vi "InitMeasurement.vi"(8 "error in (no error)":errorcluster) -> (0 "error out":errorcluster)   [LabVIEW 2015, in "ESLSCDLL.lvlib"]
uses:
  ESLSCDLL.lvlib
  Globals.vi
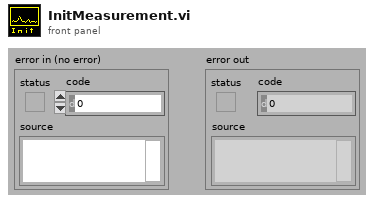
[diagram p1: front panel]
types:
  T1 = cluster{"region size[0]":u32, "region size[1]":u32, "region size[2]":u32, "region size[3]":u32, "region size[4]":u32, "region size[5]":u32, "region size[6]":u32, "region size[7]":u32}
  T2 = cluster{"dac board1[0]":u32, "dac board1[1]":u32, "dac board1[2]":u32, "dac board1[3]":u32, "dac board1[4]":u32, "dac board1[5]":u32, "dac board1[6]":u32, "dac board1[7]":u32}
  T3 = cluster{"ioctrl out width[5ns][0]":u32, "ioctrl out width[5ns][1]":u32, "ioctrl out width[5ns][2]":u32, "ioctrl out width[5ns][3]":u32, "ioctrl out width[5ns][4]":u32, "ioctrl out width[5ns][5]":u32, "ioctrl out width[5ns][6]":u32, "ioctrl out width[5ns][7]":u32}
  T4 = cluster{"ioctrl out delay[5ns][0]":u32, "ioctrl out delay[5ns][1]":u32, "ioctrl out delay[5ns][2]":u32, "ioctrl out delay[5ns][3]":u32, "ioctrl out delay[5ns][4]":u32, "ioctrl out delay[5ns][5]":u32, "ioctrl out delay[5ns][6]":u32, "ioctrl out delay[5ns][7]":u32}
  T5 = cluster{"dac board2[0]":u32, "dac board2[1]":u32, "dac board2[2]":u32, "dac board2[3]":u32, "dac board2[4]":u32, "dac board2[5]":u32, "dac board2[6]":u32, "dac board2[7]":u32}
  T6 = cluster{"[0]":u8, "[1]":u8, "[2]":u8, "[3]":u8, "[4]":u8, "[5]":u8, "[6]":u8, "[7]":u8, "[8]":u8, "[9]":u8, "[10]":u8, "[11]":u8, "[12]":u8, "[13]":u8, "[14]":u8, "[15]":u8, "[16]":u8, "[17]":u8, "[18]":u8, "[19]":u8, "[20]":u8, "[21]":u8, "[22]":u8, "[23]":u8, "[24]":u8, "[25]":u8, "[26]":u8, "[27]":u8, "[28]":u8, "[29]":u8, "[30]":u8, "[31]":u8, "[32]":u8, "[33]":u8, "[34]":u8, "[35]":u8, "[36]":u8, "[37]":u8, "[38]":u8, "[39]":u8, "[40]":u8, "[41]":u8, "[42]":u8, "[43]":u8, "[44]":u8, "[45]":u8, "[46]":u8, "[47]":u8, "[48]":u8, "[49]":u8, "[50]":u8, "[51]":u8, "[52]":u8, "[53]":u8, "[54]":u8, "[55]":u8, "[56]":u8, "[57]":u8, "[58]":u8, "[59]":u8, "[60]":u8, "[61]":u8, "[62]":u8, "[63]":u8, "[64]":u8, "[65]":u8, "[66]":u8, "[67]":u8, "[68]":u8, "[69]":u8, "[70]":u8, "[71]":u8, "[72]":u8, "[73]":u8, "[74]":u8, "[75]":u8, "[76]":u8, "[77]":u8, "[78]":u8, "[79]":u8, "[80]":u8, "[81]":u8, "[82]":u8, "[83]":u8, "[84]":u8, "[85]":u8, "[86]":u8, "[87]":u8, "[88]":u8, "[89]":u8, "[90]":u8, "[91]":u8, "[92]":u8, "[93]":u8, "[94]":u8, "[95]":u8, "[96]":u8, "[97]":u8, "[98]":u8, "[99]":u8, "[100]":u8, "[101]":u8, "[102]":u8, "[103]":u8, "[104]":u8, "[105]":u8, "[106]":u8, "[107]":u8, "[108]":u8, "[109]":u8, "[110]":u8, "[111]":u8, "[112]":u8, "[113]":u8, "[114]":u8, "[115]":u8, "[116]":u8, "[117]":u8, "[118]":u8, "[119]":u8, "[120]":u8, "[121]":u8, "[122]":u8, "[123]":u8, "[124]":u8, "[125]":u8, "[126]":u8, "[127]":u8, "[128]":u8, "[129]":u8, "[130]":u8, "[131]":u8, "[132]":u8, "[133]":u8, "[134]":u8, "[135]":u8, "[136]":u8, "[137]":u8, "[138]":u8, "[139]":u8, "[140]":u8, "[141]":u8, "[142]":u8, "[143]":u8, "[144]":u8, "[145]":u8, "[146]":u8, "[147]":u8, "[148]":u8, "[149]":u8, "[150]":u8, "[151]":u8, "[152]":u8, "[153]":u8, "[154]":u8, "[155]":u8, "[156]":u8, "[157]":u8, "[158]":u8, "[159]":u8, "[160]":u8, "[161]":u8, "[162]":u8, "[163]":u8, "[164]":u8, "[165]":u8, "[166]":u8, "[167]":u8, "[168]":u8, "[169]":u8, "[170]":u8, "[171]":u8, "[172]":u8, "[173]":u8, "[174]":u8, "[175]":u8, "[176]":u8, "[177]":u8, "[178]":u8, "[179]":u8, "[180]":u8, "[181]":u8, "[182]":u8, "[183]":u8, "[184]":u8, "[185]":u8, "[186]":u8, "[187]":u8, "[188]":u8, "[189]":u8, "[190]":u8, "[191]":u8, "[192]":u8, "[193]":u8, "[194]":u8, "[195]":u8, "[196]":u8, "[197]":u8, "[198]":u8, "[199]":u8, "[200]":u8, "[201]":u8, "[202]":u8, "[203]":u8, "[204]":u8, "[205]":u8, "[206]":u8, "[207]":u8, "[208]":u8, "[209]":u8, "[210]":u8, "[211]":u8, "[212]":u8, "[213]":u8, "[214]":u8, "[215]":u8, "[216]":u8, "[217]":u8, "[218]":u8, "[219]":u8, "[220]":u8, "[221]":u8, "[222]":u8, "[223]":u8, "[224]":u8, "[225]":u8, "[226]":u8, "[227]":u8, "[228]":u8, "[229]":u8, "[230]":u8, "[231]":u8, "[232]":u8, "[233]":u8, "[234]":u8, "[235]":u8, "[236]":u8, "[237]":u8, "[238]":u8, "[239]":u8, "[240]":u8, "[241]":u8, "[242]":u8, "[243]":u8, "[244]":u8, "[245]":u8, "[246]":u8, "[247]":u8, "[248]":u8, "[249]":u8, "[250]":u8, "[251]":u8, "[252]":u8, "[253]":u8, "[254]":u8, "[255]":u8}
  T7 = cluster{"dac board3[0]":u32, "dac board3[1]":u32, "dac board3[2]":u32, "dac board3[3]":u32, "dac board3[4]":u32, "dac board3[5]":u32, "dac board3[6]":u32, "dac board3[7]":u32}
  T8 = cluster{"dac board4[0]":u32, "dac board4[1]":u32, "dac board4[2]":u32, "dac board4[3]":u32, "dac board4[4]":u32, "dac board4[5]":u32, "dac board4[6]":u32, "dac board4[7]":u32}
  T9 = cluster{"dac board5[0]":u32, "dac board5[1]":u32, "dac board5[2]":u32, "dac board5[3]":u32, "dac board5[4]":u32, "dac board5[5]":u32, "dac board5[6]":u32, "dac board5[7]":u32}
  T10 = enum32{"Full Binning", "Region of Interest", "Area"}
  T11 = enum32{"XCK", "Reg/OutTrig", "VON", "DMA_Act", "ASLS", "STIMER", "BTIMER", "INTRSR", "S1", "S2", "BON", "MEASUREON", "SDAT", "BDAT", "SSHUT", "BSHUT", "IFC", "DO_CC_I", "EXPOSURE_WINDOW", "TO_CNT_OUT", "SECON", "I", "unused2", "unused3", "unused4", "unused5", "unused6", "unused7", "unused8", "ENFFR", "ENFFW", "ENFFWRPROT"}
  T12 = enum32{"I", "S1", "S2", "S1&S2", "BTimer", "S1 chopper", "S2 chopper", "S1&S2 chopper"}
  T13 = enum32{"I", "S1", "S2", "S2=EN_I", "STimer", "ASL"}
  T14 = cluster{u32, "sti":enum32{"I", "S1", "S2", "S2=EN_I", "STimer", "ASL"}, "bti":enum32{"I", "S1", "S2", "S1&S2", "BTimer", "S1 chopper", "S2 chopper", "S1&S2 chopper"}, u32, u32, "sdat in 10ns":u32, "bdat in 10ns":u32, "st slope":enum32{"pos", "neg", "both"}, "bt slope":enum32{"neg", "pos", "both"}, "xckdly in 10ns":u32, "sec in 10ns":u32, "cc trigger":enum32{"XCK", "Ext. Trig.", "DAT"}, u32, "CAMERA SYSTEM":u32, "CAMCNT":u32, "PIXEL":u32, u32, u32, "sensor gain":u32, "adc gain":u32, "cool level":u32, u32, "gpx offset":u32, "LINES":u32, "VFREQ":u32, "fft mode":enum32{"Full Binning", "Region of Interest", "Area"}, "area lines binning":u32, "nor":u32, u8, "region size":cluster{"region size[0]":u32, "region size[1]":u32, "region size[2]":u32, "region size[3]":u32, "region size[4]":u32, "region size[5]":u32, "region size[6]":u32, "region size[7]":u32}, "dac board1":cluster{"dac board1[0]":u32, "dac board1[1]":u32, "dac board1[2]":u32, "dac board1[3]":u32, "dac board1[4]":u32, "dac board1[5]":u32, "dac board1[6]":u32, "dac board1[7]":u32}, "tor":enum32{"XCK", "Reg/OutTrig", "VON", "DMA_Act", "ASLS", "STIMER", "BTIMER", "INTRSR", "S1", "S2", "BON", "MEASUREON", "SDAT", "BDAT", "SSHUT", "BSHUT", "IFC", "DO_CC_I", "EXPOSURE_WINDOW", "TO_CNT_OUT", "SECON", "I", "unused2", "unused3", "unused4", "unused5", "unused6", "unused7", "unused8", "ENFFR", "ENFFW", "ENFFWRPROT"}, "adc mode":enum16{"normal", "ramp", "custom pattern"}, "custom pattern":u32, "bec in 10\nns":u32, u32, "ioctrl impact start pixel":u32, "ioctrl out width[5ns]":cluster{"ioctrl out width[5ns][0]":u32, "ioctrl out width[5ns][1]":u32, "ioctrl out width[5ns][2]":u32, "ioctrl out width[5ns][3]":u32, "ioctrl out width[5ns][4]":u32, "ioctrl out width[5ns][5]":u32, "ioctrl out width[5ns][6]":u32, "ioctrl out width[5ns][7]":u32}, "ioctrl out delay[5ns]":cluster{"ioctrl out delay[5ns][0]":u32, "ioctrl out delay[5ns][1]":u32, "ioctrl out delay[5ns][2]":u32, "ioctrl out delay[5ns][3]":u32, "ioctrl out delay[5ns][4]":u32, "ioctrl out delay[5ns][5]":u32, "ioctrl out delay[5ns][6]":u32, "ioctrl out delay[5ns][7]":u32}, "ioctrl t0 period[10ns]":u32, "dma buffer size in scans":u32, "tocnt":u32, "ticnt":u32, u32, u32, cluster{"[0]":u8, "[1]":u8, "[2]":u8, "[3]":u8, "[4]":u8, "[5]":u8, "[6]":u8, "[7]":u8, "[8]":u8, "[9]":u8, "[10]":u8, "[11]":u8, "[12]":u8, "[13]":u8, "[14]":u8, "[15]":u8, "[16]":u8, "[17]":u8, "[18]":u8, "[19]":u8, "[20]":u8, "[21]":u8, "[22]":u8, "[23]":u8, "[24]":u8, "[25]":u8, "[26]":u8, "[27]":u8, "[28]":u8, "[29]":u8, "[30]":u8, "[31]":u8, "[32]":u8, "[33]":u8, "[34]":u8, "[35]":u8, "[36]":u8, "[37]":u8, "[38]":u8, "[39]":u8, "[40]":u8, "[41]":u8, "[42]":u8, "[43]":u8, "[44]":u8, "[45]":u8, "[46]":u8, "[47]":u8, "[48]":u8, "[49]":u8, "[50]":u8, "[51]":u8, "[52]":u8, "[53]":u8, "[54]":u8, "[55]":u8, "[56]":u8, "[57]":u8, "[58]":u8, "[59]":u8, "[60]":u8, "[61]":u8, "[62]":u8, "[63]":u8, "[64]":u8, "[65]":u8, "[66]":u8, "[67]":u8, "[68]":u8, "[69]":u8, "[70]":u8, "[71]":u8, "[72]":u8, "[73]":u8, "[74]":u8, "[75]":u8, "[76]":u8, "[77]":u8, "[78]":u8, "[79]":u8, "[80]":u8, "[81]":u8, "[82]":u8, "[83]":u8, "[84]":u8, "[85]":u8, "[86]":u8, "[87]":u8, "[88]":u8, "[89]":u8, "[90]":u8, "[91]":u8, "[92]":u8, "[93]":u8, "[94]":u8, "[95]":u8, "[96]":u8, "[97]":u8, "[98]":u8, "[99]":u8, "[100]":u8, "[101]":u8, "[102]":u8, "[103]":u8, "[104]":u8, "[105]":u8, "[106]":u8, "[107]":u8, "[108]":u8, "[109]":u8, "[110]":u8, "[111]":u8, "[112]":u8, "[113]":u8, "[114]":u8, "[115]":u8, "[116]":u8, "[117]":u8, "[118]":u8, "[119]":u8, "[120]":u8, "[121]":u8, "[122]":u8, "[123]":u8, "[124]":u8, "[125]":u8, "[126]":u8, "[127]":u8, "[128]":u8, "[129]":u8, "[130]":u8, "[131]":u8, "[132]":u8, "[133]":u8, "[134]":u8, "[135]":u8, "[136]":u8, "[137]":u8, "[138]":u8, "[139]":u8, "[140]":u8, "[141]":u8, "[142]":u8, "[143]":u8, "[144]":u8, "[145]":u8, "[146]":u8, "[147]":u8, "[148]":u8, "[149]":u8, "[150]":u8, "[151]":u8, "[152]":u8, "[153]":u8, "[154]":u8, "[155]":u8, "[156]":u8, "[157]":u8, "[158]":u8, "[159]":u8, "[160]":u8, "[161]":u8, "[162]":u8, "[163]":u8, "[164]":u8, "[165]":u8, "[166]":u8, "[167]":u8, "[168]":u8, "[169]":u8, "[170]":u8, "[171]":u8, "[172]":u8, "[173]":u8, "[174]":u8, "[175]":u8, "[176]":u8, "[177]":u8, "[178]":u8, "[179]":u8, "[180]":u8, "[181]":u8, "[182]":u8, "[183]":u8, "[184]":u8, "[185]":u8, "[186]":u8, "[187]":u8, "[188]":u8, "[189]":u8, "[190]":u8, "[191]":u8, "[192]":u8, "[193]":u8, "[194]":u8, "[195]":u8, "[196]":u8, "[197]":u8, "[198]":u8, "[199]":u8, "[200]":u8, "[201]":u8, "[202]":u8, "[203]":u8, "[204]":u8, "[205]":u8, "[206]":u8, "[207]":u8, "[208]":u8, "[209]":u8, "[210]":u8, "[211]":u8, "[212]":u8, "[213]":u8, "[214]":u8, "[215]":u8, "[216]":u8, "[217]":u8, "[218]":u8, "[219]":u8, "[220]":u8, "[221]":u8, "[222]":u8, "[223]":u8, "[224]":u8, "[225]":u8, "[226]":u8, "[227]":u8, "[228]":u8, "[229]":u8, "[230]":u8, "[231]":u8, "[232]":u8, "[233]":u8, "[234]":u8, "[235]":u8, "[236]":u8, "[237]":u8, "[238]":u8, "[239]":u8, "[240]":u8, "[241]":u8, "[242]":u8, "[243]":u8, "[244]":u8, "[245]":u8, "[246]":u8, "[247]":u8, "[248]":u8, "[249]":u8, "[250]":u8, "[251]":u8, "[252]":u8, "[253]":u8, "[254]":u8, "[255]":u8}, "unused (deprecated file split mode)":u32, u32}
  T15 = cluster{u32, "sti":enum32{"I", "S1", "S2", "S2=EN_I", "STimer", "ASL"}, "bti":enum32{"I", "S1", "S2", "S1&S2", "BTimer", "S1 chopper", "S2 chopper", "S1&S2 chopper"}, u32, u32, "sdat in 10ns":u32, "bdat in 10ns":u32, "st slope":enum32{"pos", "neg", "both"}, "bt slope":enum32{"neg", "pos", "both"}, "xckdly in 10ns":u32, "sec in 10ns":u32, "cc trigger":enum32{"XCK", "Ext. Trig.", "DAT"}, u32, "CAMERA SYSTEM":u32, "CAMCNT":u32, "PIXEL":u32, u32, u32, "sensor gain":u32, "adc gain":u32, "cool level":u32, u32, "gpx offset":u32, "LINES":u32, "VFREQ":u32, "fft mode":enum32{"Full Binning", "Region of Interest", "Area"}, "area lines binning":u32, "nor":u32, u8, "region size":cluster{"region size[0]":u32, "region size[1]":u32, "region size[2]":u32, "region size[3]":u32, "region size[4]":u32, "region size[5]":u32, "region size[6]":u32, "region size[7]":u32}, "dac board2":cluster{"dac board2[0]":u32, "dac board2[1]":u32, "dac board2[2]":u32, "dac board2[3]":u32, "dac board2[4]":u32, "dac board2[5]":u32, "dac board2[6]":u32, "dac board2[7]":u32}, "tor":enum32{"XCK", "Reg/OutTrig", "VON", "DMA_Act", "ASLS", "STIMER", "BTIMER", "INTRSR", "S1", "S2", "BON", "MEASUREON", "SDAT", "BDAT", "SSHUT", "BSHUT", "IFC", "DO_CC_I", "EXPOSURE_WINDOW", "TO_CNT_OUT", "SECON", "I", "unused2", "unused3", "unused4", "unused5", "unused6", "unused7", "unused8", "ENFFR", "ENFFW", "ENFFWRPROT"}, "adc mode":enum16{"normal", "ramp", "custom pattern"}, "custom pattern":u32, "bec in 10\nns":u32, u32, "ioctrl impact start pixel":u32, "ioctrl out width[5ns]":cluster{"ioctrl out width[5ns][0]":u32, "ioctrl out width[5ns][1]":u32, "ioctrl out width[5ns][2]":u32, "ioctrl out width[5ns][3]":u32, "ioctrl out width[5ns][4]":u32, "ioctrl out width[5ns][5]":u32, "ioctrl out width[5ns][6]":u32, "ioctrl out width[5ns][7]":u32}, "ioctrl out delay[5ns]":cluster{"ioctrl out delay[5ns][0]":u32, "ioctrl out delay[5ns][1]":u32, "ioctrl out delay[5ns][2]":u32, "ioctrl out delay[5ns][3]":u32, "ioctrl out delay[5ns][4]":u32, "ioctrl out delay[5ns][5]":u32, "ioctrl out delay[5ns][6]":u32, "ioctrl out delay[5ns][7]":u32}, "ioctrl t0 period[10ns]":u32, "dma buffer size in scans":u32, "tocnt":u32, "ticnt":u32, u32, u32, cluster{"[0]":u8, "[1]":u8, "[2]":u8, "[3]":u8, "[4]":u8, "[5]":u8, "[6]":u8, "[7]":u8, "[8]":u8, "[9]":u8, "[10]":u8, "[11]":u8, "[12]":u8, "[13]":u8, "[14]":u8, "[15]":u8, "[16]":u8, "[17]":u8, "[18]":u8, "[19]":u8, "[20]":u8, "[21]":u8, "[22]":u8, "[23]":u8, "[24]":u8, "[25]":u8, "[26]":u8, "[27]":u8, "[28]":u8, "[29]":u8, "[30]":u8, "[31]":u8, "[32]":u8, "[33]":u8, "[34]":u8, "[35]":u8, "[36]":u8, "[37]":u8, "[38]":u8, "[39]":u8, "[40]":u8, "[41]":u8, "[42]":u8, "[43]":u8, "[44]":u8, "[45]":u8, "[46]":u8, "[47]":u8, "[48]":u8, "[49]":u8, "[50]":u8, "[51]":u8, "[52]":u8, "[53]":u8, "[54]":u8, "[55]":u8, "[56]":u8, "[57]":u8, "[58]":u8, "[59]":u8, "[60]":u8, "[61]":u8, "[62]":u8, "[63]":u8, "[64]":u8, "[65]":u8, "[66]":u8, "[67]":u8, "[68]":u8, "[69]":u8, "[70]":u8, "[71]":u8, "[72]":u8, "[73]":u8, "[74]":u8, "[75]":u8, "[76]":u8, "[77]":u8, "[78]":u8, "[79]":u8, "[80]":u8, "[81]":u8, "[82]":u8, "[83]":u8, "[84]":u8, "[85]":u8, "[86]":u8, "[87]":u8, "[88]":u8, "[89]":u8, "[90]":u8, "[91]":u8, "[92]":u8, "[93]":u8, "[94]":u8, "[95]":u8, "[96]":u8, "[97]":u8, "[98]":u8, "[99]":u8, "[100]":u8, "[101]":u8, "[102]":u8, "[103]":u8, "[104]":u8, "[105]":u8, "[106]":u8, "[107]":u8, "[108]":u8, "[109]":u8, "[110]":u8, "[111]":u8, "[112]":u8, "[113]":u8, "[114]":u8, "[115]":u8, "[116]":u8, "[117]":u8, "[118]":u8, "[119]":u8, "[120]":u8, "[121]":u8, "[122]":u8, "[123]":u8, "[124]":u8, "[125]":u8, "[126]":u8, "[127]":u8, "[128]":u8, "[129]":u8, "[130]":u8, "[131]":u8, "[132]":u8, "[133]":u8, "[134]":u8, "[135]":u8, "[136]":u8, "[137]":u8, "[138]":u8, "[139]":u8, "[140]":u8, "[141]":u8, "[142]":u8, "[143]":u8, "[144]":u8, "[145]":u8, "[146]":u8, "[147]":u8, "[148]":u8, "[149]":u8, "[150]":u8, "[151]":u8, "[152]":u8, "[153]":u8, "[154]":u8, "[155]":u8, "[156]":u8, "[157]":u8, "[158]":u8, "[159]":u8, "[160]":u8, "[161]":u8, "[162]":u8, "[163]":u8, "[164]":u8, "[165]":u8, "[166]":u8, "[167]":u8, "[168]":u8, "[169]":u8, "[170]":u8, "[171]":u8, "[172]":u8, "[173]":u8, "[174]":u8, "[175]":u8, "[176]":u8, "[177]":u8, "[178]":u8, "[179]":u8, "[180]":u8, "[181]":u8, "[182]":u8, "[183]":u8, "[184]":u8, "[185]":u8, "[186]":u8, "[187]":u8, "[188]":u8, "[189]":u8, "[190]":u8, "[191]":u8, "[192]":u8, "[193]":u8, "[194]":u8, "[195]":u8, "[196]":u8, "[197]":u8, "[198]":u8, "[199]":u8, "[200]":u8, "[201]":u8, "[202]":u8, "[203]":u8, "[204]":u8, "[205]":u8, "[206]":u8, "[207]":u8, "[208]":u8, "[209]":u8, "[210]":u8, "[211]":u8, "[212]":u8, "[213]":u8, "[214]":u8, "[215]":u8, "[216]":u8, "[217]":u8, "[218]":u8, "[219]":u8, "[220]":u8, "[221]":u8, "[222]":u8, "[223]":u8, "[224]":u8, "[225]":u8, "[226]":u8, "[227]":u8, "[228]":u8, "[229]":u8, "[230]":u8, "[231]":u8, "[232]":u8, "[233]":u8, "[234]":u8, "[235]":u8, "[236]":u8, "[237]":u8, "[238]":u8, "[239]":u8, "[240]":u8, "[241]":u8, "[242]":u8, "[243]":u8, "[244]":u8, "[245]":u8, "[246]":u8, "[247]":u8, "[248]":u8, "[249]":u8, "[250]":u8, "[251]":u8, "[252]":u8, "[253]":u8, "[254]":u8, "[255]":u8}, "unused (deprecated file split mode)":u32, u32}
  T16 = cluster{u32, "sti":enum32{"I", "S1", "S2", "S2=EN_I", "STimer", "ASL"}, "bti":enum32{"I", "S1", "S2", "S1&S2", "BTimer", "S1 chopper", "S2 chopper", "S1&S2 chopper"}, u32, u32, "sdat in 10ns":u32, "bdat in 10ns":u32, "st slope":enum32{"pos", "neg", "both"}, "bt slope":enum32{"neg", "pos", "both"}, "xckdly in 10ns":u32, "sec in 10ns":u32, "cc trigger":enum32{"XCK", "Ext. Trig.", "DAT"}, u32, "CAMERA SYSTEM":u32, "CAMCNT":u32, "PIXEL":u32, u32, u32, "sensor gain":u32, "adc gain":u32, "cool level":u32, u32, "gpx offset":u32, "LINES":u32, "VFREQ":u32, "fft mode":enum32{"Full Binning", "Region of Interest", "Area"}, "area lines binning":u32, "nor":u32, u8, "region size":cluster{"region size[0]":u32, "region size[1]":u32, "region size[2]":u32, "region size[3]":u32, "region size[4]":u32, "region size[5]":u32, "region size[6]":u32, "region size[7]":u32}, "dac board3":cluster{"dac board3[0]":u32, "dac board3[1]":u32, "dac board3[2]":u32, "dac board3[3]":u32, "dac board3[4]":u32, "dac board3[5]":u32, "dac board3[6]":u32, "dac board3[7]":u32}, "tor":enum32{"XCK", "Reg/OutTrig", "VON", "DMA_Act", "ASLS", "STIMER", "BTIMER", "INTRSR", "S1", "S2", "BON", "MEASUREON", "SDAT", "BDAT", "SSHUT", "BSHUT", "IFC", "DO_CC_I", "EXPOSURE_WINDOW", "TO_CNT_OUT", "SECON", "I", "unused2", "unused3", "unused4", "unused5", "unused6", "unused7", "unused8", "ENFFR", "ENFFW", "ENFFWRPROT"}, "adc mode":enum16{"normal", "ramp", "custom pattern"}, "custom pattern":u32, "bec in 10\nns":u32, u32, "ioctrl impact start pixel":u32, "ioctrl out width[5ns]":cluster{"ioctrl out width[5ns][0]":u32, "ioctrl out width[5ns][1]":u32, "ioctrl out width[5ns][2]":u32, "ioctrl out width[5ns][3]":u32, "ioctrl out width[5ns][4]":u32, "ioctrl out width[5ns][5]":u32, "ioctrl out width[5ns][6]":u32, "ioctrl out width[5ns][7]":u32}, "ioctrl out delay[5ns]":cluster{"ioctrl out delay[5ns][0]":u32, "ioctrl out delay[5ns][1]":u32, "ioctrl out delay[5ns][2]":u32, "ioctrl out delay[5ns][3]":u32, "ioctrl out delay[5ns][4]":u32, "ioctrl out delay[5ns][5]":u32, "ioctrl out delay[5ns][6]":u32, "ioctrl out delay[5ns][7]":u32}, "ioctrl t0 period[10ns]":u32, "dma buffer size in scans":u32, "tocnt":u32, "ticnt":u32, u32, u32, cluster{"[0]":u8, "[1]":u8, "[2]":u8, "[3]":u8, "[4]":u8, "[5]":u8, "[6]":u8, "[7]":u8, "[8]":u8, "[9]":u8, "[10]":u8, "[11]":u8, "[12]":u8, "[13]":u8, "[14]":u8, "[15]":u8, "[16]":u8, "[17]":u8, "[18]":u8, "[19]":u8, "[20]":u8, "[21]":u8, "[22]":u8, "[23]":u8, "[24]":u8, "[25]":u8, "[26]":u8, "[27]":u8, "[28]":u8, "[29]":u8, "[30]":u8, "[31]":u8, "[32]":u8, "[33]":u8, "[34]":u8, "[35]":u8, "[36]":u8, "[37]":u8, "[38]":u8, "[39]":u8, "[40]":u8, "[41]":u8, "[42]":u8, "[43]":u8, "[44]":u8, "[45]":u8, "[46]":u8, "[47]":u8, "[48]":u8, "[49]":u8, "[50]":u8, "[51]":u8, "[52]":u8, "[53]":u8, "[54]":u8, "[55]":u8, "[56]":u8, "[57]":u8, "[58]":u8, "[59]":u8, "[60]":u8, "[61]":u8, "[62]":u8, "[63]":u8, "[64]":u8, "[65]":u8, "[66]":u8, "[67]":u8, "[68]":u8, "[69]":u8, "[70]":u8, "[71]":u8, "[72]":u8, "[73]":u8, "[74]":u8, "[75]":u8, "[76]":u8, "[77]":u8, "[78]":u8, "[79]":u8, "[80]":u8, "[81]":u8, "[82]":u8, "[83]":u8, "[84]":u8, "[85]":u8, "[86]":u8, "[87]":u8, "[88]":u8, "[89]":u8, "[90]":u8, "[91]":u8, "[92]":u8, "[93]":u8, "[94]":u8, "[95]":u8, "[96]":u8, "[97]":u8, "[98]":u8, "[99]":u8, "[100]":u8, "[101]":u8, "[102]":u8, "[103]":u8, "[104]":u8, "[105]":u8, "[106]":u8, "[107]":u8, "[108]":u8, "[109]":u8, "[110]":u8, "[111]":u8, "[112]":u8, "[113]":u8, "[114]":u8, "[115]":u8, "[116]":u8, "[117]":u8, "[118]":u8, "[119]":u8, "[120]":u8, "[121]":u8, "[122]":u8, "[123]":u8, "[124]":u8, "[125]":u8, "[126]":u8, "[127]":u8, "[128]":u8, "[129]":u8, "[130]":u8, "[131]":u8, "[132]":u8, "[133]":u8, "[134]":u8, "[135]":u8, "[136]":u8, "[137]":u8, "[138]":u8, "[139]":u8, "[140]":u8, "[141]":u8, "[142]":u8, "[143]":u8, "[144]":u8, "[145]":u8, "[146]":u8, "[147]":u8, "[148]":u8, "[149]":u8, "[150]":u8, "[151]":u8, "[152]":u8, "[153]":u8, "[154]":u8, "[155]":u8, "[156]":u8, "[157]":u8, "[158]":u8, "[159]":u8, "[160]":u8, "[161]":u8, "[162]":u8, "[163]":u8, "[164]":u8, "[165]":u8, "[166]":u8, "[167]":u8, "[168]":u8, "[169]":u8, "[170]":u8, "[171]":u8, "[172]":u8, "[173]":u8, "[174]":u8, "[175]":u8, "[176]":u8, "[177]":u8, "[178]":u8, "[179]":u8, "[180]":u8, "[181]":u8, "[182]":u8, "[183]":u8, "[184]":u8, "[185]":u8, "[186]":u8, "[187]":u8, "[188]":u8, "[189]":u8, "[190]":u8, "[191]":u8, "[192]":u8, "[193]":u8, "[194]":u8, "[195]":u8, "[196]":u8, "[197]":u8, "[198]":u8, "[199]":u8, "[200]":u8, "[201]":u8, "[202]":u8, "[203]":u8, "[204]":u8, "[205]":u8, "[206]":u8, "[207]":u8, "[208]":u8, "[209]":u8, "[210]":u8, "[211]":u8, "[212]":u8, "[213]":u8, "[214]":u8, "[215]":u8, "[216]":u8, "[217]":u8, "[218]":u8, "[219]":u8, "[220]":u8, "[221]":u8, "[222]":u8, "[223]":u8, "[224]":u8, "[225]":u8, "[226]":u8, "[227]":u8, "[228]":u8, "[229]":u8, "[230]":u8, "[231]":u8, "[232]":u8, "[233]":u8, "[234]":u8, "[235]":u8, "[236]":u8, "[237]":u8, "[238]":u8, "[239]":u8, "[240]":u8, "[241]":u8, "[242]":u8, "[243]":u8, "[244]":u8, "[245]":u8, "[246]":u8, "[247]":u8, "[248]":u8, "[249]":u8, "[250]":u8, "[251]":u8, "[252]":u8, "[253]":u8, "[254]":u8, "[255]":u8}, "unused (deprecated file split mode)":u32, u32}
  T17 = cluster{u32, "sti":enum32{"I", "S1", "S2", "S2=EN_I", "STimer", "ASL"}, "bti":enum32{"I", "S1", "S2", "S1&S2", "BTimer", "S1 chopper", "S2 chopper", "S1&S2 chopper"}, u32, u32, "sdat in 10ns":u32, "bdat in 10ns":u32, "st slope":enum32{"pos", "neg", "both"}, "bt slope":enum32{"neg", "pos", "both"}, "xckdly in 10ns":u32, "sec in 10ns":u32, "cc trigger":enum32{"XCK", "Ext. Trig.", "DAT"}, u32, "CAMERA SYSTEM":u32, "CAMCNT":u32, "PIXEL":u32, u32, u32, "sensor gain":u32, "adc gain":u32, "cool level":u32, u32, "gpx offset":u32, "LINES":u32, "VFREQ":u32, "fft mode":enum32{"Full Binning", "Region of Interest", "Area"}, "area lines binning":u32, "nor":u32, u8, "region size":cluster{"region size[0]":u32, "region size[1]":u32, "region size[2]":u32, "region size[3]":u32, "region size[4]":u32, "region size[5]":u32, "region size[6]":u32, "region size[7]":u32}, "dac board4":cluster{"dac board4[0]":u32, "dac board4[1]":u32, "dac board4[2]":u32, "dac board4[3]":u32, "dac board4[4]":u32, "dac board4[5]":u32, "dac board4[6]":u32, "dac board4[7]":u32}, "tor":enum32{"XCK", "Reg/OutTrig", "VON", "DMA_Act", "ASLS", "STIMER", "BTIMER", "INTRSR", "S1", "S2", "BON", "MEASUREON", "SDAT", "BDAT", "SSHUT", "BSHUT", "IFC", "DO_CC_I", "EXPOSURE_WINDOW", "TO_CNT_OUT", "SECON", "I", "unused2", "unused3", "unused4", "unused5", "unused6", "unused7", "unused8", "ENFFR", "ENFFW", "ENFFWRPROT"}, "adc mode":enum16{"normal", "ramp", "custom pattern"}, "custom pattern":u32, "bec in 10\nns":u32, u32, "ioctrl impact start pixel":u32, "ioctrl out width[5ns]":cluster{"ioctrl out width[5ns][0]":u32, "ioctrl out width[5ns][1]":u32, "ioctrl out width[5ns][2]":u32, "ioctrl out width[5ns][3]":u32, "ioctrl out width[5ns][4]":u32, "ioctrl out width[5ns][5]":u32, "ioctrl out width[5ns][6]":u32, "ioctrl out width[5ns][7]":u32}, "ioctrl out delay[5ns]":cluster{"ioctrl out delay[5ns][0]":u32, "ioctrl out delay[5ns][1]":u32, "ioctrl out delay[5ns][2]":u32, "ioctrl out delay[5ns][3]":u32, "ioctrl out delay[5ns][4]":u32, "ioctrl out delay[5ns][5]":u32, "ioctrl out delay[5ns][6]":u32, "ioctrl out delay[5ns][7]":u32}, "ioctrl t0 period[10ns]":u32, "dma buffer size in scans":u32, "tocnt":u32, "ticnt":u32, u32, u32, cluster{"[0]":u8, "[1]":u8, "[2]":u8, "[3]":u8, "[4]":u8, "[5]":u8, "[6]":u8, "[7]":u8, "[8]":u8, "[9]":u8, "[10]":u8, "[11]":u8, "[12]":u8, "[13]":u8, "[14]":u8, "[15]":u8, "[16]":u8, "[17]":u8, "[18]":u8, "[19]":u8, "[20]":u8, "[21]":u8, "[22]":u8, "[23]":u8, "[24]":u8, "[25]":u8, "[26]":u8, "[27]":u8, "[28]":u8, "[29]":u8, "[30]":u8, "[31]":u8, "[32]":u8, "[33]":u8, "[34]":u8, "[35]":u8, "[36]":u8, "[37]":u8, "[38]":u8, "[39]":u8, "[40]":u8, "[41]":u8, "[42]":u8, "[43]":u8, "[44]":u8, "[45]":u8, "[46]":u8, "[47]":u8, "[48]":u8, "[49]":u8, "[50]":u8, "[51]":u8, "[52]":u8, "[53]":u8, "[54]":u8, "[55]":u8, "[56]":u8, "[57]":u8, "[58]":u8, "[59]":u8, "[60]":u8, "[61]":u8, "[62]":u8, "[63]":u8, "[64]":u8, "[65]":u8, "[66]":u8, "[67]":u8, "[68]":u8, "[69]":u8, "[70]":u8, "[71]":u8, "[72]":u8, "[73]":u8, "[74]":u8, "[75]":u8, "[76]":u8, "[77]":u8, "[78]":u8, "[79]":u8, "[80]":u8, "[81]":u8, "[82]":u8, "[83]":u8, "[84]":u8, "[85]":u8, "[86]":u8, "[87]":u8, "[88]":u8, "[89]":u8, "[90]":u8, "[91]":u8, "[92]":u8, "[93]":u8, "[94]":u8, "[95]":u8, "[96]":u8, "[97]":u8, "[98]":u8, "[99]":u8, "[100]":u8, "[101]":u8, "[102]":u8, "[103]":u8, "[104]":u8, "[105]":u8, "[106]":u8, "[107]":u8, "[108]":u8, "[109]":u8, "[110]":u8, "[111]":u8, "[112]":u8, "[113]":u8, "[114]":u8, "[115]":u8, "[116]":u8, "[117]":u8, "[118]":u8, "[119]":u8, "[120]":u8, "[121]":u8, "[122]":u8, "[123]":u8, "[124]":u8, "[125]":u8, "[126]":u8, "[127]":u8, "[128]":u8, "[129]":u8, "[130]":u8, "[131]":u8, "[132]":u8, "[133]":u8, "[134]":u8, "[135]":u8, "[136]":u8, "[137]":u8, "[138]":u8, "[139]":u8, "[140]":u8, "[141]":u8, "[142]":u8, "[143]":u8, "[144]":u8, "[145]":u8, "[146]":u8, "[147]":u8, "[148]":u8, "[149]":u8, "[150]":u8, "[151]":u8, "[152]":u8, "[153]":u8, "[154]":u8, "[155]":u8, "[156]":u8, "[157]":u8, "[158]":u8, "[159]":u8, "[160]":u8, "[161]":u8, "[162]":u8, "[163]":u8, "[164]":u8, "[165]":u8, "[166]":u8, "[167]":u8, "[168]":u8, "[169]":u8, "[170]":u8, "[171]":u8, "[172]":u8, "[173]":u8, "[174]":u8, "[175]":u8, "[176]":u8, "[177]":u8, "[178]":u8, "[179]":u8, "[180]":u8, "[181]":u8, "[182]":u8, "[183]":u8, "[184]":u8, "[185]":u8, "[186]":u8, "[187]":u8, "[188]":u8, "[189]":u8, "[190]":u8, "[191]":u8, "[192]":u8, "[193]":u8, "[194]":u8, "[195]":u8, "[196]":u8, "[197]":u8, "[198]":u8, "[199]":u8, "[200]":u8, "[201]":u8, "[202]":u8, "[203]":u8, "[204]":u8, "[205]":u8, "[206]":u8, "[207]":u8, "[208]":u8, "[209]":u8, "[210]":u8, "[211]":u8, "[212]":u8, "[213]":u8, "[214]":u8, "[215]":u8, "[216]":u8, "[217]":u8, "[218]":u8, "[219]":u8, "[220]":u8, "[221]":u8, "[222]":u8, "[223]":u8, "[224]":u8, "[225]":u8, "[226]":u8, "[227]":u8, "[228]":u8, "[229]":u8, "[230]":u8, "[231]":u8, "[232]":u8, "[233]":u8, "[234]":u8, "[235]":u8, "[236]":u8, "[237]":u8, "[238]":u8, "[239]":u8, "[240]":u8, "[241]":u8, "[242]":u8, "[243]":u8, "[244]":u8, "[245]":u8, "[246]":u8, "[247]":u8, "[248]":u8, "[249]":u8, "[250]":u8, "[251]":u8, "[252]":u8, "[253]":u8, "[254]":u8, "[255]":u8}, "unused (deprecated file split mode)":u32, u32}
  T18 = cluster{u32, "sti":enum32{"I", "S1", "S2", "S2=EN_I", "STimer", "ASL"}, "bti":enum32{"I", "S1", "S2", "S1&S2", "BTimer", "S1 chopper", "S2 chopper", "S1&S2 chopper"}, u32, u32, "sdat in 10ns":u32, "bdat in 10ns":u32, "st slope":enum32{"pos", "neg", "both"}, "bt slope":enum32{"neg", "pos", "both"}, "xckdly in 10ns":u32, "sec in 10ns":u32, "cc trigger":enum32{"XCK", "Ext. Trig.", "DAT"}, u32, "CAMERA SYSTEM":u32, "CAMCNT":u32, "PIXEL":u32, u32, u32, "sensor gain":u32, "adc gain":u32, "cool level":u32, u32, "gpx offset":u32, "LINES":u32, "VFREQ":u32, "fft mode":enum32{"Full Binning", "Region of Interest", "Area"}, "area lines binning":u32, "nor":u32, u8, "region size":cluster{"region size[0]":u32, "region size[1]":u32, "region size[2]":u32, "region size[3]":u32, "region size[4]":u32, "region size[5]":u32, "region size[6]":u32, "region size[7]":u32}, "dac board5":cluster{"dac board5[0]":u32, "dac board5[1]":u32, "dac board5[2]":u32, "dac board5[3]":u32, "dac board5[4]":u32, "dac board5[5]":u32, "dac board5[6]":u32, "dac board5[7]":u32}, "tor":enum32{"XCK", "Reg/OutTrig", "VON", "DMA_Act", "ASLS", "STIMER", "BTIMER", "INTRSR", "S1", "S2", "BON", "MEASUREON", "SDAT", "BDAT", "SSHUT", "BSHUT", "IFC", "DO_CC_I", "EXPOSURE_WINDOW", "TO_CNT_OUT", "SECON", "I", "unused2", "unused3", "unused4", "unused5", "unused6", "unused7", "unused8", "ENFFR", "ENFFW", "ENFFWRPROT"}, "adc mode":enum16{"normal", "ramp", "custom pattern"}, "custom pattern":u32, "bec in 10\nns":u32, u32, "ioctrl impact start pixel":u32, "ioctrl out width[5ns]":cluster{"ioctrl out width[5ns][0]":u32, "ioctrl out width[5ns][1]":u32, "ioctrl out width[5ns][2]":u32, "ioctrl out width[5ns][3]":u32, "ioctrl out width[5ns][4]":u32, "ioctrl out width[5ns][5]":u32, "ioctrl out width[5ns][6]":u32, "ioctrl out width[5ns][7]":u32}, "ioctrl out delay[5ns]":cluster{"ioctrl out delay[5ns][0]":u32, "ioctrl out delay[5ns][1]":u32, "ioctrl out delay[5ns][2]":u32, "ioctrl out delay[5ns][3]":u32, "ioctrl out delay[5ns][4]":u32, "ioctrl out delay[5ns][5]":u32, "ioctrl out delay[5ns][6]":u32, "ioctrl out delay[5ns][7]":u32}, "ioctrl t0 period[10ns]":u32, "dma buffer size in scans":u32, "tocnt":u32, "ticnt":u32, u32, u32, cluster{"[0]":u8, "[1]":u8, "[2]":u8, "[3]":u8, "[4]":u8, "[5]":u8, "[6]":u8, "[7]":u8, "[8]":u8, "[9]":u8, "[10]":u8, "[11]":u8, "[12]":u8, "[13]":u8, "[14]":u8, "[15]":u8, "[16]":u8, "[17]":u8, "[18]":u8, "[19]":u8, "[20]":u8, "[21]":u8, "[22]":u8, "[23]":u8, "[24]":u8, "[25]":u8, "[26]":u8, "[27]":u8, "[28]":u8, "[29]":u8, "[30]":u8, "[31]":u8, "[32]":u8, "[33]":u8, "[34]":u8, "[35]":u8, "[36]":u8, "[37]":u8, "[38]":u8, "[39]":u8, "[40]":u8, "[41]":u8, "[42]":u8, "[43]":u8, "[44]":u8, "[45]":u8, "[46]":u8, "[47]":u8, "[48]":u8, "[49]":u8, "[50]":u8, "[51]":u8, "[52]":u8, "[53]":u8, "[54]":u8, "[55]":u8, "[56]":u8, "[57]":u8, "[58]":u8, "[59]":u8, "[60]":u8, "[61]":u8, "[62]":u8, "[63]":u8, "[64]":u8, "[65]":u8, "[66]":u8, "[67]":u8, "[68]":u8, "[69]":u8, "[70]":u8, "[71]":u8, "[72]":u8, "[73]":u8, "[74]":u8, "[75]":u8, "[76]":u8, "[77]":u8, "[78]":u8, "[79]":u8, "[80]":u8, "[81]":u8, "[82]":u8, "[83]":u8, "[84]":u8, "[85]":u8, "[86]":u8, "[87]":u8, "[88]":u8, "[89]":u8, "[90]":u8, "[91]":u8, "[92]":u8, "[93]":u8, "[94]":u8, "[95]":u8, "[96]":u8, "[97]":u8, "[98]":u8, "[99]":u8, "[100]":u8, "[101]":u8, "[102]":u8, "[103]":u8, "[104]":u8, "[105]":u8, "[106]":u8, "[107]":u8, "[108]":u8, "[109]":u8, "[110]":u8, "[111]":u8, "[112]":u8, "[113]":u8, "[114]":u8, "[115]":u8, "[116]":u8, "[117]":u8, "[118]":u8, "[119]":u8, "[120]":u8, "[121]":u8, "[122]":u8, "[123]":u8, "[124]":u8, "[125]":u8, "[126]":u8, "[127]":u8, "[128]":u8, "[129]":u8, "[130]":u8, "[131]":u8, "[132]":u8, "[133]":u8, "[134]":u8, "[135]":u8, "[136]":u8, "[137]":u8, "[138]":u8, "[139]":u8, "[140]":u8, "[141]":u8, "[142]":u8, "[143]":u8, "[144]":u8, "[145]":u8, "[146]":u8, "[147]":u8, "[148]":u8, "[149]":u8, "[150]":u8, "[151]":u8, "[152]":u8, "[153]":u8, "[154]":u8, "[155]":u8, "[156]":u8, "[157]":u8, "[158]":u8, "[159]":u8, "[160]":u8, "[161]":u8, "[162]":u8, "[163]":u8, "[164]":u8, "[165]":u8, "[166]":u8, "[167]":u8, "[168]":u8, "[169]":u8, "[170]":u8, "[171]":u8, "[172]":u8, "[173]":u8, "[174]":u8, "[175]":u8, "[176]":u8, "[177]":u8, "[178]":u8, "[179]":u8, "[180]":u8, "[181]":u8, "[182]":u8, "[183]":u8, "[184]":u8, "[185]":u8, "[186]":u8, "[187]":u8, "[188]":u8, "[189]":u8, "[190]":u8, "[191]":u8, "[192]":u8, "[193]":u8, "[194]":u8, "[195]":u8, "[196]":u8, "[197]":u8, "[198]":u8, "[199]":u8, "[200]":u8, "[201]":u8, "[202]":u8, "[203]":u8, "[204]":u8, "[205]":u8, "[206]":u8, "[207]":u8, "[208]":u8, "[209]":u8, "[210]":u8, "[211]":u8, "[212]":u8, "[213]":u8, "[214]":u8, "[215]":u8, "[216]":u8, "[217]":u8, "[218]":u8, "[219]":u8, "[220]":u8, "[221]":u8, "[222]":u8, "[223]":u8, "[224]":u8, "[225]":u8, "[226]":u8, "[227]":u8, "[228]":u8, "[229]":u8, "[230]":u8, "[231]":u8, "[232]":u8, "[233]":u8, "[234]":u8, "[235]":u8, "[236]":u8, "[237]":u8, "[238]":u8, "[239]":u8, "[240]":u8, "[241]":u8, "[242]":u8, "[243]":u8, "[244]":u8, "[245]":u8, "[246]":u8, "[247]":u8, "[248]":u8, "[249]":u8, "[250]":u8, "[251]":u8, "[252]":u8, "[253]":u8, "[254]":u8, "[255]":u8}, "unused (deprecated file split mode)":u32, u32}
  T19 = cluster{"board_sel":u32, "nos":u32, "nob":u32, u32, "cont pause in microseconds":u32, cluster{u32, "sti":enum32{"I", "S1", "S2", "S2=EN_I", "STimer", "ASL"}, "bti":enum32{"I", "S1", "S2", "S1&S2", "BTimer", "S1 chopper", "S2 chopper", "S1&S2 chopper"}, u32, u32, "sdat in 10ns":u32, "bdat in 10ns":u32, "st slope":enum32{"pos", "neg", "both"}, "bt slope":enum32{"neg", "pos", "both"}, "xckdly in 10ns":u32, "sec in 10ns":u32, "cc trigger":enum32{"XCK", "Ext. Trig.", "DAT"}, u32, "CAMERA SYSTEM":u32, "CAMCNT":u32, "PIXEL":u32, u32, u32, "sensor gain":u32, "adc gain":u32, "cool level":u32, u32, "gpx offset":u32, "LINES":u32, "VFREQ":u32, "fft mode":enum32{"Full Binning", "Region of Interest", "Area"}, "area lines binning":u32, "nor":u32, u8, "region size":cluster{"region size[0]":u32, "region size[1]":u32, "region size[2]":u32, "region size[3]":u32, "region size[4]":u32, "region size[5]":u32, "region size[6]":u32, "region size[7]":u32}, "dac board1":cluster{"dac board1[0]":u32, "dac board1[1]":u32, "dac board1[2]":u32, "dac board1[3]":u32, "dac board1[4]":u32, "dac board1[5]":u32, "dac board1[6]":u32, "dac board1[7]":u32}, "tor":enum32{"XCK", "Reg/OutTrig", "VON", "DMA_Act", "ASLS", "STIMER", "BTIMER", "INTRSR", "S1", "S2", "BON", "MEASUREON", "SDAT", "BDAT", "SSHUT", "BSHUT", "IFC", "DO_CC_I", "EXPOSURE_WINDOW", "TO_CNT_OUT", "SECON", "I", "unused2", "unused3", "unused4", "unused5", "unused6", "unused7", "unused8", "ENFFR", "ENFFW", "ENFFWRPROT"}, "adc mode":enum16{"normal", "ramp", "custom pattern"}, "custom pattern":u32, "bec in 10\nns":u32, u32, "ioctrl impact start pixel":u32, "ioctrl out width[5ns]":cluster{"ioctrl out width[5ns][0]":u32, "ioctrl out width[5ns][1]":u32, "ioctrl out width[5ns][2]":u32, "ioctrl out width[5ns][3]":u32, "ioctrl out width[5ns][4]":u32, "ioctrl out width[5ns][5]":u32, "ioctrl out width[5ns][6]":u32, "ioctrl out width[5ns][7]":u32}, "ioctrl out delay[5ns]":cluster{"ioctrl out delay[5ns][0]":u32, "ioctrl out delay[5ns][1]":u32, "ioctrl out delay[5ns][2]":u32, "ioctrl out delay[5ns][3]":u32, "ioctrl out delay[5ns][4]":u32, "ioctrl out delay[5ns][5]":u32, "ioctrl out delay[5ns][6]":u32, "ioctrl out delay[5ns][7]":u32}, "ioctrl t0 period[10ns]":u32, "dma buffer size in scans":u32, "tocnt":u32, "ticnt":u32, u32, u32, cluster{"[0]":u8, "[1]":u8, "[2]":u8, "[3]":u8, "[4]":u8, "[5]":u8, "[6]":u8, "[7]":u8, "[8]":u8, "[9]":u8, "[10]":u8, "[11]":u8, "[12]":u8, "[13]":u8, "[14]":u8, "[15]":u8, "[16]":u8, "[17]":u8, "[18]":u8, "[19]":u8, "[20]":u8, "[21]":u8, "[22]":u8, "[23]":u8, "[24]":u8, "[25]":u8, "[26]":u8, "[27]":u8, "[28]":u8, "[29]":u8, "[30]":u8, "[31]":u8, "[32]":u8, "[33]":u8, "[34]":u8, "[35]":u8, "[36]":u8, "[37]":u8, "[38]":u8, "[39]":u8, "[40]":u8, "[41]":u8, "[42]":u8, "[43]":u8, "[44]":u8, "[45]":u8, "[46]":u8, "[47]":u8, "[48]":u8, "[49]":u8, "[50]":u8, "[51]":u8, "[52]":u8, "[53]":u8, "[54]":u8, "[55]":u8, "[56]":u8, "[57]":u8, "[58]":u8, "[59]":u8, "[60]":u8, "[61]":u8, "[62]":u8, "[63]":u8, "[64]":u8, "[65]":u8, "[66]":u8, "[67]":u8, "[68]":u8, "[69]":u8, "[70]":u8, "[71]":u8, "[72]":u8, "[73]":u8, "[74]":u8, "[75]":u8, "[76]":u8, "[77]":u8, "[78]":u8, "[79]":u8, "[80]":u8, "[81]":u8, "[82]":u8, "[83]":u8, "[84]":u8, "[85]":u8, "[86]":u8, "[87]":u8, "[88]":u8, "[89]":u8, "[90]":u8, "[91]":u8, "[92]":u8, "[93]":u8, "[94]":u8, "[95]":u8, "[96]":u8, "[97]":u8, "[98]":u8, "[99]":u8, "[100]":u8, "[101]":u8, "[102]":u8, "[103]":u8, "[104]":u8, "[105]":u8, "[106]":u8, "[107]":u8, "[108]":u8, "[109]":u8, "[110]":u8, "[111]":u8, "[112]":u8, "[113]":u8, "[114]":u8, "[115]":u8, "[116]":u8, "[117]":u8, "[118]":u8, "[119]":u8, "[120]":u8, "[121]":u8, "[122]":u8, "[123]":u8, "[124]":u8, "[125]":u8, "[126]":u8, "[127]":u8, "[128]":u8, "[129]":u8, "[130]":u8, "[131]":u8, "[132]":u8, "[133]":u8, "[134]":u8, "[135]":u8, "[136]":u8, "[137]":u8, "[138]":u8, "[139]":u8, "[140]":u8, "[141]":u8, "[142]":u8, "[143]":u8, "[144]":u8, "[145]":u8, "[146]":u8, "[147]":u8, "[148]":u8, "[149]":u8, "[150]":u8, "[151]":u8, "[152]":u8, "[153]":u8, "[154]":u8, "[155]":u8, "[156]":u8, "[157]":u8, "[158]":u8, "[159]":u8, "[160]":u8, "[161]":u8, "[162]":u8, "[163]":u8, "[164]":u8, "[165]":u8, "[166]":u8, "[167]":u8, "[168]":u8, "[169]":u8, "[170]":u8, "[171]":u8, "[172]":u8, "[173]":u8, "[174]":u8, "[175]":u8, "[176]":u8, "[177]":u8, "[178]":u8, "[179]":u8, "[180]":u8, "[181]":u8, "[182]":u8, "[183]":u8, "[184]":u8, "[185]":u8, "[186]":u8, "[187]":u8, "[188]":u8, "[189]":u8, "[190]":u8, "[191]":u8, "[192]":u8, "[193]":u8, "[194]":u8, "[195]":u8, "[196]":u8, "[197]":u8, "[198]":u8, "[199]":u8, "[200]":u8, "[201]":u8, "[202]":u8, "[203]":u8, "[204]":u8, "[205]":u8, "[206]":u8, "[207]":u8, "[208]":u8, "[209]":u8, "[210]":u8, "[211]":u8, "[212]":u8, "[213]":u8, "[214]":u8, "[215]":u8, "[216]":u8, "[217]":u8, "[218]":u8, "[219]":u8, "[220]":u8, "[221]":u8, "[222]":u8, "[223]":u8, "[224]":u8, "[225]":u8, "[226]":u8, "[227]":u8, "[228]":u8, "[229]":u8, "[230]":u8, "[231]":u8, "[232]":u8, "[233]":u8, "[234]":u8, "[235]":u8, "[236]":u8, "[237]":u8, "[238]":u8, "[239]":u8, "[240]":u8, "[241]":u8, "[242]":u8, "[243]":u8, "[244]":u8, "[245]":u8, "[246]":u8, "[247]":u8, "[248]":u8, "[249]":u8, "[250]":u8, "[251]":u8, "[252]":u8, "[253]":u8, "[254]":u8, "[255]":u8}, "unused (deprecated file split mode)":u32, u32}, cluster{u32, "sti":enum32{"I", "S1", "S2", "S2=EN_I", "STimer", "ASL"}, "bti":enum32{"I", "S1", "S2", "S1&S2", "BTimer", "S1 chopper", "S2 chopper", "S1&S2 chopper"}, u32, u32, "sdat in 10ns":u32, "bdat in 10ns":u32, "st slope":enum32{"pos", "neg", "both"}, "bt slope":enum32{"neg", "pos", "both"}, "xckdly in 10ns":u32, "sec in 10ns":u32, "cc trigger":enum32{"XCK", "Ext. Trig.", "DAT"}, u32, "CAMERA SYSTEM":u32, "CAMCNT":u32, "PIXEL":u32, u32, u32, "sensor gain":u32, "adc gain":u32, "cool level":u32, u32, "gpx offset":u32, "LINES":u32, "VFREQ":u32, "fft mode":enum32{"Full Binning", "Region of Interest", "Area"}, "area lines binning":u32, "nor":u32, u8, "region size":cluster{"region size[0]":u32, "region size[1]":u32, "region size[2]":u32, "region size[3]":u32, "region size[4]":u32, "region size[5]":u32, "region size[6]":u32, "region size[7]":u32}, "dac board2":cluster{"dac board2[0]":u32, "dac board2[1]":u32, "dac board2[2]":u32, "dac board2[3]":u32, "dac board2[4]":u32, "dac board2[5]":u32, "dac board2[6]":u32, "dac board2[7]":u32}, "tor":enum32{"XCK", "Reg/OutTrig", "VON", "DMA_Act", "ASLS", "STIMER", "BTIMER", "INTRSR", "S1", "S2", "BON", "MEASUREON", "SDAT", "BDAT", "SSHUT", "BSHUT", "IFC", "DO_CC_I", "EXPOSURE_WINDOW", "TO_CNT_OUT", "SECON", "I", "unused2", "unused3", "unused4", "unused5", "unused6", "unused7", "unused8", "ENFFR", "ENFFW", "ENFFWRPROT"}, "adc mode":enum16{"normal", "ramp", "custom pattern"}, "custom pattern":u32, "bec in 10\nns":u32, u32, "ioctrl impact start pixel":u32, "ioctrl out width[5ns]":cluster{"ioctrl out width[5ns][0]":u32, "ioctrl out width[5ns][1]":u32, "ioctrl out width[5ns][2]":u32, "ioctrl out width[5ns][3]":u32, "ioctrl out width[5ns][4]":u32, "ioctrl out width[5ns][5]":u32, "ioctrl out width[5ns][6]":u32, "ioctrl out width[5ns][7]":u32}, "ioctrl out delay[5ns]":cluster{"ioctrl out delay[5ns][0]":u32, "ioctrl out delay[5ns][1]":u32, "ioctrl out delay[5ns][2]":u32, "ioctrl out delay[5ns][3]":u32, "ioctrl out delay[5ns][4]":u32, "ioctrl out delay[5ns][5]":u32, "ioctrl out delay[5ns][6]":u32, "ioctrl out delay[5ns][7]":u32}, "ioctrl t0 period[10ns]":u32, "dma buffer size in scans":u32, "tocnt":u32, "ticnt":u32, u32, u32, cluster{"[0]":u8, "[1]":u8, "[2]":u8, "[3]":u8, "[4]":u8, "[5]":u8, "[6]":u8, "[7]":u8, "[8]":u8, "[9]":u8, "[10]":u8, "[11]":u8, "[12]":u8, "[13]":u8, "[14]":u8, "[15]":u8, "[16]":u8, "[17]":u8, "[18]":u8, "[19]":u8, "[20]":u8, "[21]":u8, "[22]":u8, "[23]":u8, "[24]":u8, "[25]":u8, "[26]":u8, "[27]":u8, "[28]":u8, "[29]":u8, "[30]":u8, "[31]":u8, "[32]":u8, "[33]":u8, "[34]":u8, "[35]":u8, "[36]":u8, "[37]":u8, "[38]":u8, "[39]":u8, "[40]":u8, "[41]":u8, "[42]":u8, "[43]":u8, "[44]":u8, "[45]":u8, "[46]":u8, "[47]":u8, "[48]":u8, "[49]":u8, "[50]":u8, "[51]":u8, "[52]":u8, "[53]":u8, "[54]":u8, "[55]":u8, "[56]":u8, "[57]":u8, "[58]":u8, "[59]":u8, "[60]":u8, "[61]":u8, "[62]":u8, "[63]":u8, "[64]":u8, "[65]":u8, "[66]":u8, "[67]":u8, "[68]":u8, "[69]":u8, "[70]":u8, "[71]":u8, "[72]":u8, "[73]":u8, "[74]":u8, "[75]":u8, "[76]":u8, "[77]":u8, "[78]":u8, "[79]":u8, "[80]":u8, "[81]":u8, "[82]":u8, "[83]":u8, "[84]":u8, "[85]":u8, "[86]":u8, "[87]":u8, "[88]":u8, "[89]":u8, "[90]":u8, "[91]":u8, "[92]":u8, "[93]":u8, "[94]":u8, "[95]":u8, "[96]":u8, "[97]":u8, "[98]":u8, "[99]":u8, "[100]":u8, "[101]":u8, "[102]":u8, "[103]":u8, "[104]":u8, "[105]":u8, "[106]":u8, "[107]":u8, "[108]":u8, "[109]":u8, "[110]":u8, "[111]":u8, "[112]":u8, "[113]":u8, "[114]":u8, "[115]":u8, "[116]":u8, "[117]":u8, "[118]":u8, "[119]":u8, "[120]":u8, "[121]":u8, "[122]":u8, "[123]":u8, "[124]":u8, "[125]":u8, "[126]":u8, "[127]":u8, "[128]":u8, "[129]":u8, "[130]":u8, "[131]":u8, "[132]":u8, "[133]":u8, "[134]":u8, "[135]":u8, "[136]":u8, "[137]":u8, "[138]":u8, "[139]":u8, "[140]":u8, "[141]":u8, "[142]":u8, "[143]":u8, "[144]":u8, "[145]":u8, "[146]":u8, "[147]":u8, "[148]":u8, "[149]":u8, "[150]":u8, "[151]":u8, "[152]":u8, "[153]":u8, "[154]":u8, "[155]":u8, "[156]":u8, "[157]":u8, "[158]":u8, "[159]":u8, "[160]":u8, "[161]":u8, "[162]":u8, "[163]":u8, "[164]":u8, "[165]":u8, "[166]":u8, "[167]":u8, "[168]":u8, "[169]":u8, "[170]":u8, "[171]":u8, "[172]":u8, "[173]":u8, "[174]":u8, "[175]":u8, "[176]":u8, "[177]":u8, "[178]":u8, "[179]":u8, "[180]":u8, "[181]":u8, "[182]":u8, "[183]":u8, "[184]":u8, "[185]":u8, "[186]":u8, "[187]":u8, "[188]":u8, "[189]":u8, "[190]":u8, "[191]":u8, "[192]":u8, "[193]":u8, "[194]":u8, "[195]":u8, "[196]":u8, "[197]":u8, "[198]":u8, "[199]":u8, "[200]":u8, "[201]":u8, "[202]":u8, "[203]":u8, "[204]":u8, "[205]":u8, "[206]":u8, "[207]":u8, "[208]":u8, "[209]":u8, "[210]":u8, "[211]":u8, "[212]":u8, "[213]":u8, "[214]":u8, "[215]":u8, "[216]":u8, "[217]":u8, "[218]":u8, "[219]":u8, "[220]":u8, "[221]":u8, "[222]":u8, "[223]":u8, "[224]":u8, "[225]":u8, "[226]":u8, "[227]":u8, "[228]":u8, "[229]":u8, "[230]":u8, "[231]":u8, "[232]":u8, "[233]":u8, "[234]":u8, "[235]":u8, "[236]":u8, "[237]":u8, "[238]":u8, "[239]":u8, "[240]":u8, "[241]":u8, "[242]":u8, "[243]":u8, "[244]":u8, "[245]":u8, "[246]":u8, "[247]":u8, "[248]":u8, "[249]":u8, "[250]":u8, "[251]":u8, "[252]":u8, "[253]":u8, "[254]":u8, "[255]":u8}, "unused (deprecated file split mode)":u32, u32}, cluster{u32, "sti":enum32{"I", "S1", "S2", "S2=EN_I", "STimer", "ASL"}, "bti":enum32{"I", "S1", "S2", "S1&S2", "BTimer", "S1 chopper", "S2 chopper", "S1&S2 chopper"}, u32, u32, "sdat in 10ns":u32, "bdat in 10ns":u32, "st slope":enum32{"pos", "neg", "both"}, "bt slope":enum32{"neg", "pos", "both"}, "xckdly in 10ns":u32, "sec in 10ns":u32, "cc trigger":enum32{"XCK", "Ext. Trig.", "DAT"}, u32, "CAMERA SYSTEM":u32, "CAMCNT":u32, "PIXEL":u32, u32, u32, "sensor gain":u32, "adc gain":u32, "cool level":u32, u32, "gpx offset":u32, "LINES":u32, "VFREQ":u32, "fft mode":enum32{"Full Binning", "Region of Interest", "Area"}, "area lines binning":u32, "nor":u32, u8, "region size":cluster{"region size[0]":u32, "region size[1]":u32, "region size[2]":u32, "region size[3]":u32, "region size[4]":u32, "region size[5]":u32, "region size[6]":u32, "region size[7]":u32}, "dac board3":cluster{"dac board3[0]":u32, "dac board3[1]":u32, "dac board3[2]":u32, "dac board3[3]":u32, "dac board3[4]":u32, "dac board3[5]":u32, "dac board3[6]":u32, "dac board3[7]":u32}, "tor":enum32{"XCK", "Reg/OutTrig", "VON", "DMA_Act", "ASLS", "STIMER", "BTIMER", "INTRSR", "S1", "S2", "BON", "MEASUREON", "SDAT", "BDAT", "SSHUT", "BSHUT", "IFC", "DO_CC_I", "EXPOSURE_WINDOW", "TO_CNT_OUT", "SECON", "I", "unused2", "unused3", "unused4", "unused5", "unused6", "unused7", "unused8", "ENFFR", "ENFFW", "ENFFWRPROT"}, "adc mode":enum16{"normal", "ramp", "custom pattern"}, "custom pattern":u32, "bec in 10\nns":u32, u32, "ioctrl impact start pixel":u32, "ioctrl out width[5ns]":cluster{"ioctrl out width[5ns][0]":u32, "ioctrl out width[5ns][1]":u32, "ioctrl out width[5ns][2]":u32, "ioctrl out width[5ns][3]":u32, "ioctrl out width[5ns][4]":u32, "ioctrl out width[5ns][5]":u32, "ioctrl out width[5ns][6]":u32, "ioctrl out width[5ns][7]":u32}, "ioctrl out delay[5ns]":cluster{"ioctrl out delay[5ns][0]":u32, "ioctrl out delay[5ns][1]":u32, "ioctrl out delay[5ns][2]":u32, "ioctrl out delay[5ns][3]":u32, "ioctrl out delay[5ns][4]":u32, "ioctrl out delay[5ns][5]":u32, "ioctrl out delay[5ns][6]":u32, "ioctrl out delay[5ns][7]":u32}, "ioctrl t0 period[10ns]":u32, "dma buffer size in scans":u32, "tocnt":u32, "ticnt":u32, u32, u32, cluster{"[0]":u8, "[1]":u8, "[2]":u8, "[3]":u8, "[4]":u8, "[5]":u8, "[6]":u8, "[7]":u8, "[8]":u8, "[9]":u8, "[10]":u8, "[11]":u8, "[12]":u8, "[13]":u8, "[14]":u8, "[15]":u8, "[16]":u8, "[17]":u8, "[18]":u8, "[19]":u8, "[20]":u8, "[21]":u8, "[22]":u8, "[23]":u8, "[24]":u8, "[25]":u8, "[26]":u8, "[27]":u8, "[28]":u8, "[29]":u8, "[30]":u8, "[31]":u8, "[32]":u8, "[33]":u8, "[34]":u8, "[35]":u8, "[36]":u8, "[37]":u8, "[38]":u8, "[39]":u8, "[40]":u8, "[41]":u8, "[42]":u8, "[43]":u8, "[44]":u8, "[45]":u8, "[46]":u8, "[47]":u8, "[48]":u8, "[49]":u8, "[50]":u8, "[51]":u8, "[52]":u8, "[53]":u8, "[54]":u8, "[55]":u8, "[56]":u8, "[57]":u8, "[58]":u8, "[59]":u8, "[60]":u8, "[61]":u8, "[62]":u8, "[63]":u8, "[64]":u8, "[65]":u8, "[66]":u8, "[67]":u8, "[68]":u8, "[69]":u8, "[70]":u8, "[71]":u8, "[72]":u8, "[73]":u8, "[74]":u8, "[75]":u8, "[76]":u8, "[77]":u8, "[78]":u8, "[79]":u8, "[80]":u8, "[81]":u8, "[82]":u8, "[83]":u8, "[84]":u8, "[85]":u8, "[86]":u8, "[87]":u8, "[88]":u8, "[89]":u8, "[90]":u8, "[91]":u8, "[92]":u8, "[93]":u8, "[94]":u8, "[95]":u8, "[96]":u8, "[97]":u8, "[98]":u8, "[99]":u8, "[100]":u8, "[101]":u8, "[102]":u8, "[103]":u8, "[104]":u8, "[105]":u8, "[106]":u8, "[107]":u8, "[108]":u8, "[109]":u8, "[110]":u8, "[111]":u8, "[112]":u8, "[113]":u8, "[114]":u8, "[115]":u8, "[116]":u8, "[117]":u8, "[118]":u8, "[119]":u8, "[120]":u8, "[121]":u8, "[122]":u8, "[123]":u8, "[124]":u8, "[125]":u8, "[126]":u8, "[127]":u8, "[128]":u8, "[129]":u8, "[130]":u8, "[131]":u8, "[132]":u8, "[133]":u8, "[134]":u8, "[135]":u8, "[136]":u8, "[137]":u8, "[138]":u8, "[139]":u8, "[140]":u8, "[141]":u8, "[142]":u8, "[143]":u8, "[144]":u8, "[145]":u8, "[146]":u8, "[147]":u8, "[148]":u8, "[149]":u8, "[150]":u8, "[151]":u8, "[152]":u8, "[153]":u8, "[154]":u8, "[155]":u8, "[156]":u8, "[157]":u8, "[158]":u8, "[159]":u8, "[160]":u8, "[161]":u8, "[162]":u8, "[163]":u8, "[164]":u8, "[165]":u8, "[166]":u8, "[167]":u8, "[168]":u8, "[169]":u8, "[170]":u8, "[171]":u8, "[172]":u8, "[173]":u8, "[174]":u8, "[175]":u8, "[176]":u8, "[177]":u8, "[178]":u8, "[179]":u8, "[180]":u8, "[181]":u8, "[182]":u8, "[183]":u8, "[184]":u8, "[185]":u8, "[186]":u8, "[187]":u8, "[188]":u8, "[189]":u8, "[190]":u8, "[191]":u8, "[192]":u8, "[193]":u8, "[194]":u8, "[195]":u8, "[196]":u8, "[197]":u8, "[198]":u8, "[199]":u8, "[200]":u8, "[201]":u8, "[202]":u8, "[203]":u8, "[204]":u8, "[205]":u8, "[206]":u8, "[207]":u8, "[208]":u8, "[209]":u8, "[210]":u8, "[211]":u8, "[212]":u8, "[213]":u8, "[214]":u8, "[215]":u8, "[216]":u8, "[217]":u8, "[218]":u8, "[219]":u8, "[220]":u8, "[221]":u8, "[222]":u8, "[223]":u8, "[224]":u8, "[225]":u8, "[226]":u8, "[227]":u8, "[228]":u8, "[229]":u8, "[230]":u8, "[231]":u8, "[232]":u8, "[233]":u8, "[234]":u8, "[235]":u8, "[236]":u8, "[237]":u8, "[238]":u8, "[239]":u8, "[240]":u8, "[241]":u8, "[242]":u8, "[243]":u8, "[244]":u8, "[245]":u8, "[246]":u8, "[247]":u8, "[248]":u8, "[249]":u8, "[250]":u8, "[251]":u8, "[252]":u8, "[253]":u8, "[254]":u8, "[255]":u8}, "unused (deprecated file split mode)":u32, u32}, cluster{u32, "sti":enum32{"I", "S1", "S2", "S2=EN_I", "STimer", "ASL"}, "bti":enum32{"I", "S1", "S2", "S1&S2", "BTimer", "S1 chopper", "S2 chopper", "S1&S2 chopper"}, u32, u32, "sdat in 10ns":u32, "bdat in 10ns":u32, "st slope":enum32{"pos", "neg", "both"}, "bt slope":enum32{"neg", "pos", "both"}, "xckdly in 10ns":u32, "sec in 10ns":u32, "cc trigger":enum32{"XCK", "Ext. Trig.", "DAT"}, u32, "CAMERA SYSTEM":u32, "CAMCNT":u32, "PIXEL":u32, u32, u32, "sensor gain":u32, "adc gain":u32, "cool level":u32, u32, "gpx offset":u32, "LINES":u32, "VFREQ":u32, "fft mode":enum32{"Full Binning", "Region of Interest", "Area"}, "area lines binning":u32, "nor":u32, u8, "region size":cluster{"region size[0]":u32, "region size[1]":u32, "region size[2]":u32, "region size[3]":u32, "region size[4]":u32, "region size[5]":u32, "region size[6]":u32, "region size[7]":u32}, "dac board4":cluster{"dac board4[0]":u32, "dac board4[1]":u32, "dac board4[2]":u32, "dac board4[3]":u32, "dac board4[4]":u32, "dac board4[5]":u32, "dac board4[6]":u32, "dac board4[7]":u32}, "tor":enum32{"XCK", "Reg/OutTrig", "VON", "DMA_Act", "ASLS", "STIMER", "BTIMER", "INTRSR", "S1", "S2", "BON", "MEASUREON", "SDAT", "BDAT", "SSHUT", "BSHUT", "IFC", "DO_CC_I", "EXPOSURE_WINDOW", "TO_CNT_OUT", "SECON", "I", "unused2", "unused3", "unused4", "unused5", "unused6", "unused7", "unused8", "ENFFR", "ENFFW", "ENFFWRPROT"}, "adc mode":enum16{"normal", "ramp", "custom pattern"}, "custom pattern":u32, "bec in 10\nns":u32, u32, "ioctrl impact start pixel":u32, "ioctrl out width[5ns]":cluster{"ioctrl out width[5ns][0]":u32, "ioctrl out width[5ns][1]":u32, "ioctrl out width[5ns][2]":u32, "ioctrl out width[5ns][3]":u32, "ioctrl out width[5ns][4]":u32, "ioctrl out width[5ns][5]":u32, "ioctrl out width[5ns][6]":u32, "ioctrl out width[5ns][7]":u32}, "ioctrl out delay[5ns]":cluster{"ioctrl out delay[5ns][0]":u32, "ioctrl out delay[5ns][1]":u32, "ioctrl out delay[5ns][2]":u32, "ioctrl out delay[5ns][3]":u32, "ioctrl out delay[5ns][4]":u32, "ioctrl out delay[5ns][5]":u32, "ioctrl out delay[5ns][6]":u32, "ioctrl out delay[5ns][7]":u32}, "ioctrl t0 period[10ns]":u32, "dma buffer size in scans":u32, "tocnt":u32, "ticnt":u32, u32, u32, cluster{"[0]":u8, "[1]":u8, "[2]":u8, "[3]":u8, "[4]":u8, "[5]":u8, "[6]":u8, "[7]":u8, "[8]":u8, "[9]":u8, "[10]":u8, "[11]":u8, "[12]":u8, "[13]":u8, "[14]":u8, "[15]":u8, "[16]":u8, "[17]":u8, "[18]":u8, "[19]":u8, "[20]":u8, "[21]":u8, "[22]":u8, "[23]":u8, "[24]":u8, "[25]":u8, "[26]":u8, "[27]":u8, "[28]":u8, "[29]":u8, "[30]":u8, "[31]":u8, "[32]":u8, "[33]":u8, "[34]":u8, "[35]":u8, "[36]":u8, "[37]":u8, "[38]":u8, "[39]":u8, "[40]":u8, "[41]":u8, "[42]":u8, "[43]":u8, "[44]":u8, "[45]":u8, "[46]":u8, "[47]":u8, "[48]":u8, "[49]":u8, "[50]":u8, "[51]":u8, "[52]":u8, "[53]":u8, "[54]":u8, "[55]":u8, "[56]":u8, "[57]":u8, "[58]":u8, "[59]":u8, "[60]":u8, "[61]":u8, "[62]":u8, "[63]":u8, "[64]":u8, "[65]":u8, "[66]":u8, "[67]":u8, "[68]":u8, "[69]":u8, "[70]":u8, "[71]":u8, "[72]":u8, "[73]":u8, "[74]":u8, "[75]":u8, "[76]":u8, "[77]":u8, "[78]":u8, "[79]":u8, "[80]":u8, "[81]":u8, "[82]":u8, "[83]":u8, "[84]":u8, "[85]":u8, "[86]":u8, "[87]":u8, "[88]":u8, "[89]":u8, "[90]":u8, "[91]":u8, "[92]":u8, "[93]":u8, "[94]":u8, "[95]":u8, "[96]":u8, "[97]":u8, "[98]":u8, "[99]":u8, "[100]":u8, "[101]":u8, "[102]":u8, "[103]":u8, "[104]":u8, "[105]":u8, "[106]":u8, "[107]":u8, "[108]":u8, "[109]":u8, "[110]":u8, "[111]":u8, "[112]":u8, "[113]":u8, "[114]":u8, "[115]":u8, "[116]":u8, "[117]":u8, "[118]":u8, "[119]":u8, "[120]":u8, "[121]":u8, "[122]":u8, "[123]":u8, "[124]":u8, "[125]":u8, "[126]":u8, "[127]":u8, "[128]":u8, "[129]":u8, "[130]":u8, "[131]":u8, "[132]":u8, "[133]":u8, "[134]":u8, "[135]":u8, "[136]":u8, "[137]":u8, "[138]":u8, "[139]":u8, "[140]":u8, "[141]":u8, "[142]":u8, "[143]":u8, "[144]":u8, "[145]":u8, "[146]":u8, "[147]":u8, "[148]":u8, "[149]":u8, "[150]":u8, "[151]":u8, "[152]":u8, "[153]":u8, "[154]":u8, "[155]":u8, "[156]":u8, "[157]":u8, "[158]":u8, "[159]":u8, "[160]":u8, "[161]":u8, "[162]":u8, "[163]":u8, "[164]":u8, "[165]":u8, "[166]":u8, "[167]":u8, "[168]":u8, "[169]":u8, "[170]":u8, "[171]":u8, "[172]":u8, "[173]":u8, "[174]":u8, "[175]":u8, "[176]":u8, "[177]":u8, "[178]":u8, "[179]":u8, "[180]":u8, "[181]":u8, "[182]":u8, "[183]":u8, "[184]":u8, "[185]":u8, "[186]":u8, "[187]":u8, "[188]":u8, "[189]":u8, "[190]":u8, "[191]":u8, "[192]":u8, "[193]":u8, "[194]":u8, "[195]":u8, "[196]":u8, "[197]":u8, "[198]":u8, "[199]":u8, "[200]":u8, "[201]":u8, "[202]":u8, "[203]":u8, "[204]":u8, "[205]":u8, "[206]":u8, "[207]":u8, "[208]":u8, "[209]":u8, "[210]":u8, "[211]":u8, "[212]":u8, "[213]":u8, "[214]":u8, "[215]":u8, "[216]":u8, "[217]":u8, "[218]":u8, "[219]":u8, "[220]":u8, "[221]":u8, "[222]":u8, "[223]":u8, "[224]":u8, "[225]":u8, "[226]":u8, "[227]":u8, "[228]":u8, "[229]":u8, "[230]":u8, "[231]":u8, "[232]":u8, "[233]":u8, "[234]":u8, "[235]":u8, "[236]":u8, "[237]":u8, "[238]":u8, "[239]":u8, "[240]":u8, "[241]":u8, "[242]":u8, "[243]":u8, "[244]":u8, "[245]":u8, "[246]":u8, "[247]":u8, "[248]":u8, "[249]":u8, "[250]":u8, "[251]":u8, "[252]":u8, "[253]":u8, "[254]":u8, "[255]":u8}, "unused (deprecated file split mode)":u32, u32}, cluster{u32, "sti":enum32{"I", "S1", "S2", "S2=EN_I", "STimer", "ASL"}, "bti":enum32{"I", "S1", "S2", "S1&S2", "BTimer", "S1 chopper", "S2 chopper", "S1&S2 chopper"}, u32, u32, "sdat in 10ns":u32, "bdat in 10ns":u32, "st slope":enum32{"pos", "neg", "both"}, "bt slope":enum32{"neg", "pos", "both"}, "xckdly in 10ns":u32, "sec in 10ns":u32, "cc trigger":enum32{"XCK", "Ext. Trig.", "DAT"}, u32, "CAMERA SYSTEM":u32, "CAMCNT":u32, "PIXEL":u32, u32, u32, "sensor gain":u32, "adc gain":u32, "cool level":u32, u32, "gpx offset":u32, "LINES":u32, "VFREQ":u32, "fft mode":enum32{"Full Binning", "Region of Interest", "Area"}, "area lines binning":u32, "nor":u32, u8, "region size":cluster{"region size[0]":u32, "region size[1]":u32, "region size[2]":u32, "region size[3]":u32, "region size[4]":u32, "region size[5]":u32, "region size[6]":u32, "region size[7]":u32}, "dac board5":cluster{"dac board5[0]":u32, "dac board5[1]":u32, "dac board5[2]":u32, "dac board5[3]":u32, "dac board5[4]":u32, "dac board5[5]":u32, "dac board5[6]":u32, "dac board5[7]":u32}, "tor":enum32{"XCK", "Reg/OutTrig", "VON", "DMA_Act", "ASLS", "STIMER", "BTIMER", "INTRSR", "S1", "S2", "BON", "MEASUREON", "SDAT", "BDAT", "SSHUT", "BSHUT", "IFC", "DO_CC_I", "EXPOSURE_WINDOW", "TO_CNT_OUT", "SECON", "I", "unused2", "unused3", "unused4", "unused5", "unused6", "unused7", "unused8", "ENFFR", "ENFFW", "ENFFWRPROT"}, "adc mode":enum16{"normal", "ramp", "custom pattern"}, "custom pattern":u32, "bec in 10\nns":u32, u32, "ioctrl impact start pixel":u32, "ioctrl out width[5ns]":cluster{"ioctrl out width[5ns][0]":u32, "ioctrl out width[5ns][1]":u32, "ioctrl out width[5ns][2]":u32, "ioctrl out width[5ns][3]":u32, "ioctrl out width[5ns][4]":u32, "ioctrl out width[5ns][5]":u32, "ioctrl out width[5ns][6]":u32, "ioctrl out width[5ns][7]":u32}, "ioctrl out delay[5ns]":cluster{"ioctrl out delay[5ns][0]":u32, "ioctrl out delay[5ns][1]":u32, "ioctrl out delay[5ns][2]":u32, "ioctrl out delay[5ns][3]":u32, "ioctrl out delay[5ns][4]":u32, "ioctrl out delay[5ns][5]":u32, "ioctrl out delay[5ns][6]":u32, "ioctrl out delay[5ns][7]":u32}, "ioctrl t0 period[10ns]":u32, "dma buffer size in scans":u32, "tocnt":u32, "ticnt":u32, u32, u32, cluster{"[0]":u8, "[1]":u8, "[2]":u8, "[3]":u8, "[4]":u8, "[5]":u8, "[6]":u8, "[7]":u8, "[8]":u8, "[9]":u8, "[10]":u8, "[11]":u8, "[12]":u8, "[13]":u8, "[14]":u8, "[15]":u8, "[16]":u8, "[17]":u8, "[18]":u8, "[19]":u8, "[20]":u8, "[21]":u8, "[22]":u8, "[23]":u8, "[24]":u8, "[25]":u8, "[26]":u8, "[27]":u8, "[28]":u8, "[29]":u8, "[30]":u8, "[31]":u8, "[32]":u8, "[33]":u8, "[34]":u8, "[35]":u8, "[36]":u8, "[37]":u8, "[38]":u8, "[39]":u8, "[40]":u8, "[41]":u8, "[42]":u8, "[43]":u8, "[44]":u8, "[45]":u8, "[46]":u8, "[47]":u8, "[48]":u8, "[49]":u8, "[50]":u8, "[51]":u8, "[52]":u8, "[53]":u8, "[54]":u8, "[55]":u8, "[56]":u8, "[57]":u8, "[58]":u8, "[59]":u8, "[60]":u8, "[61]":u8, "[62]":u8, "[63]":u8, "[64]":u8, "[65]":u8, "[66]":u8, "[67]":u8, "[68]":u8, "[69]":u8, "[70]":u8, "[71]":u8, "[72]":u8, "[73]":u8, "[74]":u8, "[75]":u8, "[76]":u8, "[77]":u8, "[78]":u8, "[79]":u8, "[80]":u8, "[81]":u8, "[82]":u8, "[83]":u8, "[84]":u8, "[85]":u8, "[86]":u8, "[87]":u8, "[88]":u8, "[89]":u8, "[90]":u8, "[91]":u8, "[92]":u8, "[93]":u8, "[94]":u8, "[95]":u8, "[96]":u8, "[97]":u8, "[98]":u8, "[99]":u8, "[100]":u8, "[101]":u8, "[102]":u8, "[103]":u8, "[104]":u8, "[105]":u8, "[106]":u8, "[107]":u8, "[108]":u8, "[109]":u8, "[110]":u8, "[111]":u8, "[112]":u8, "[113]":u8, "[114]":u8, "[115]":u8, "[116]":u8, "[117]":u8, "[118]":u8, "[119]":u8, "[120]":u8, "[121]":u8, "[122]":u8, "[123]":u8, "[124]":u8, "[125]":u8, "[126]":u8, "[127]":u8, "[128]":u8, "[129]":u8, "[130]":u8, "[131]":u8, "[132]":u8, "[133]":u8, "[134]":u8, "[135]":u8, "[136]":u8, "[137]":u8, "[138]":u8, "[139]":u8, "[140]":u8, "[141]":u8, "[142]":u8, "[143]":u8, "[144]":u8, "[145]":u8, "[146]":u8, "[147]":u8, "[148]":u8, "[149]":u8, "[150]":u8, "[151]":u8, "[152]":u8, "[153]":u8, "[154]":u8, "[155]":u8, "[156]":u8, "[157]":u8, "[158]":u8, "[159]":u8, "[160]":u8, "[161]":u8, "[162]":u8, "[163]":u8, "[164]":u8, "[165]":u8, "[166]":u8, "[167]":u8, "[168]":u8, "[169]":u8, "[170]":u8, "[171]":u8, "[172]":u8, "[173]":u8, "[174]":u8, "[175]":u8, "[176]":u8, "[177]":u8, "[178]":u8, "[179]":u8, "[180]":u8, "[181]":u8, "[182]":u8, "[183]":u8, "[184]":u8, "[185]":u8, "[186]":u8, "[187]":u8, "[188]":u8, "[189]":u8, "[190]":u8, "[191]":u8, "[192]":u8, "[193]":u8, "[194]":u8, "[195]":u8, "[196]":u8, "[197]":u8, "[198]":u8, "[199]":u8, "[200]":u8, "[201]":u8, "[202]":u8, "[203]":u8, "[204]":u8, "[205]":u8, "[206]":u8, "[207]":u8, "[208]":u8, "[209]":u8, "[210]":u8, "[211]":u8, "[212]":u8, "[213]":u8, "[214]":u8, "[215]":u8, "[216]":u8, "[217]":u8, "[218]":u8, "[219]":u8, "[220]":u8, "[221]":u8, "[222]":u8, "[223]":u8, "[224]":u8, "[225]":u8, "[226]":u8, "[227]":u8, "[228]":u8, "[229]":u8, "[230]":u8, "[231]":u8, "[232]":u8, "[233]":u8, "[234]":u8, "[235]":u8, "[236]":u8, "[237]":u8, "[238]":u8, "[239]":u8, "[240]":u8, "[241]":u8, "[242]":u8, "[243]":u8, "[244]":u8, "[245]":u8, "[246]":u8, "[247]":u8, "[248]":u8, "[249]":u8, "[250]":u8, "[251]":u8, "[252]":u8, "[253]":u8, "[254]":u8, "[255]":u8}, "unused (deprecated file split mode)":u32, u32}}
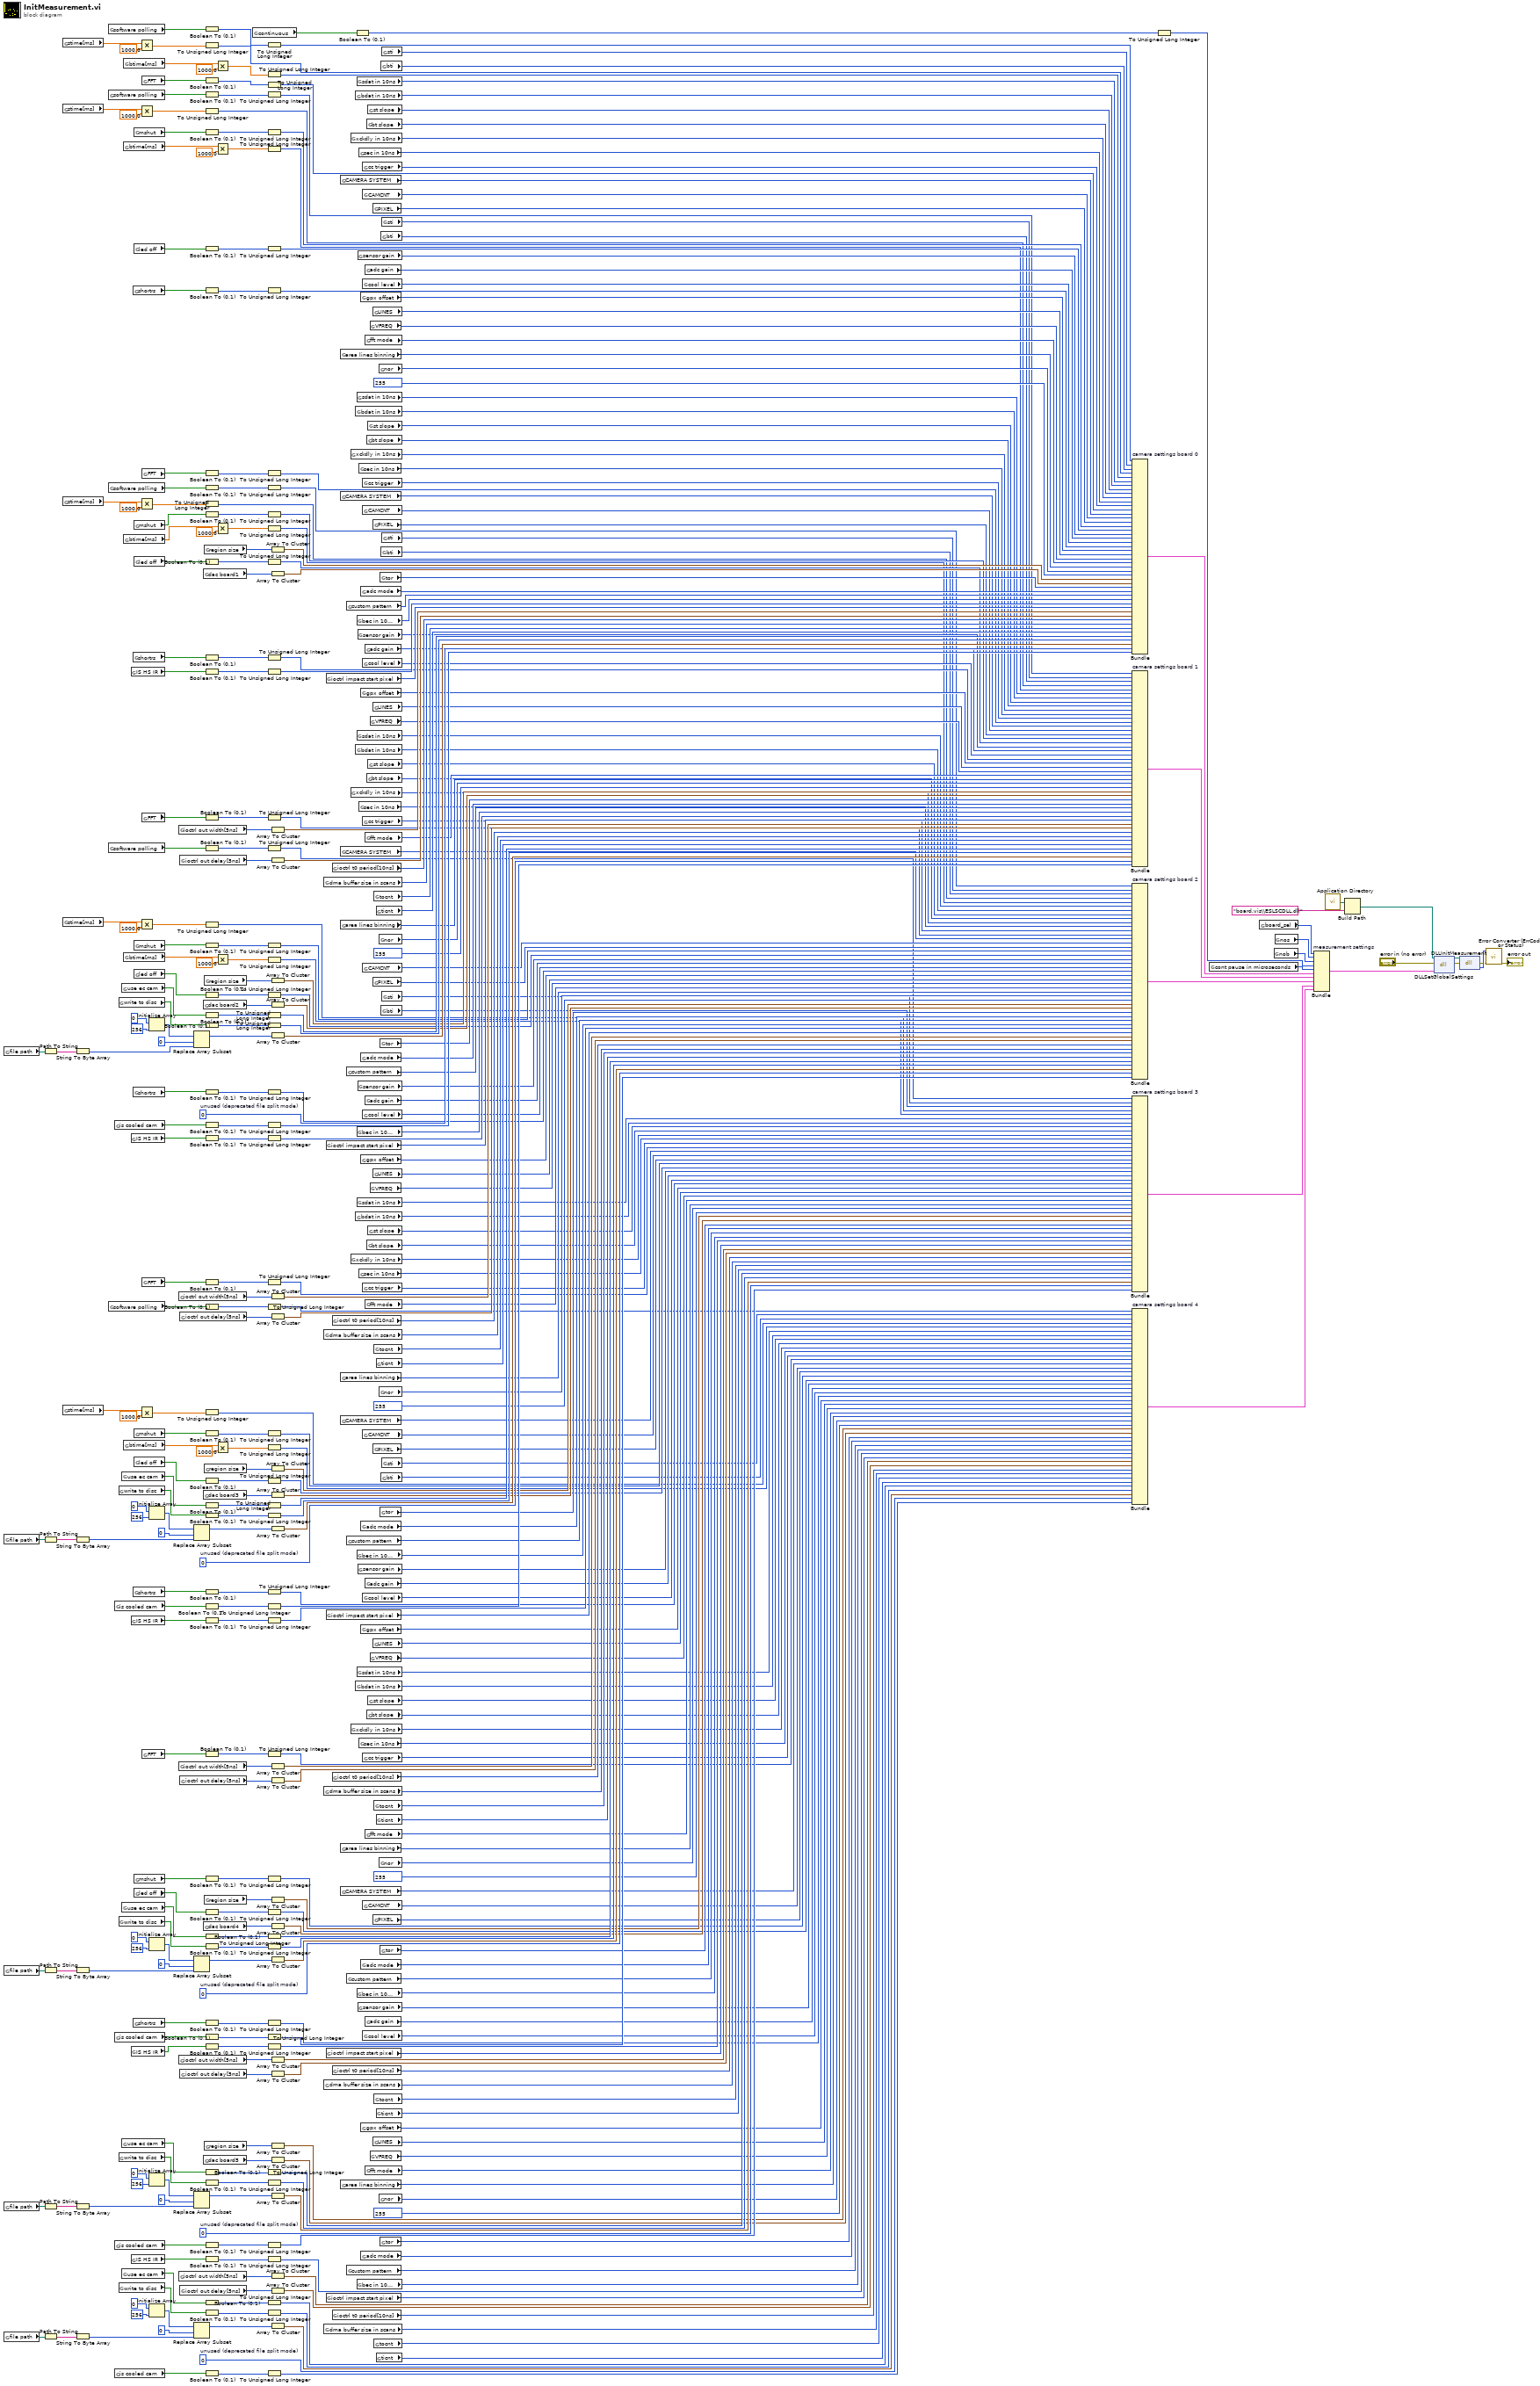
[diagram p0: block diagram]
diagram:
  w4 = u32 0  # unused (deprecated file split mode)
  w88 = u32 0  # unused (deprecated file split mode)
  w172 = u32 0  # unused (deprecated file split mode)
  w260 = u32 0  # unused (deprecated file split mode)
  w344 = u32 0  # unused (deprecated file split mode)
  n1 = global read "Globals.vi" "file path"() -> (w356:path)
  n2 = global read "Globals.vi" "file path"() -> (w272:path)
  n3 = global read "Globals.vi" "file path"() -> (w184:path)
  n4 = global read "Globals.vi" "file path"() -> (w100:path)
  n5 = global read "Globals.vi" "file path"() -> (w16:path)
  n6 = Path To String(path=w356) -> (string=w355:string)
  n7 = Path To String(path=w272) -> (string=w271:string)
  n8 = Path To String(path=w184) -> (string=w183:string)
  n9 = Path To String(path=w100) -> (string=w99:string)
  n10 = Path To String(path=w16) -> (string=w15:string)
  n11 = global read "Globals.vi" "stime[ms]"() -> (w425:dbl)
  n12 = global read "Globals.vi" "stime[ms]"() -> (w341:dbl)
  n13 = global read "Globals.vi" "stime[ms]"() -> (w253:dbl)
  n14 = global read "Globals.vi" "stime[ms]"() -> (w169:dbl)
  n15 = global read "Globals.vi" "stime[ms]"() -> (w85:dbl)
  n16 = String To Byte Array(string=w355) -> (unsigned byte array=w350:u8[])
  n17 = String To Byte Array(string=w271) -> (unsigned byte array=w266:u8[])
  n18 = String To Byte Array(string=w183) -> (unsigned byte array=w178:u8[])
  n19 = String To Byte Array(string=w99) -> (unsigned byte array=w94:u8[])
  n20 = String To Byte Array(string=w15) -> (unsigned byte array=w10:u8[])
  n21 = global read "Globals.vi" "software polling"() -> (w414:bool)
  n22 = global read "Globals.vi" "software polling"() -> (w330:bool)
  n23 = global read "Globals.vi" "software polling"() -> (w242:bool)
  n24 = global read "Globals.vi" "software polling"() -> (w158:bool)
  n25 = global read "Globals.vi" "software polling"() -> (w74:bool)
  n26 = global read "Globals.vi" "is cooled cam"() -> (w347:bool)
  n27 = global read "Globals.vi" "is cooled cam"() -> (w263:bool)
  n28 = global read "Globals.vi" "is cooled cam"() -> (w175:bool)
  n29 = global read "Globals.vi" "is cooled cam"() -> (w91:bool)
  n30 = global read "Globals.vi" "is cooled cam"() -> (w7:bool)
  n31 = global read "Globals.vi" "write to disc"() -> (w358:bool)
  n32 = global read "Globals.vi" "write to disc"() -> (w274:bool)
  n33 = global read "Globals.vi" "write to disc"() -> (w186:bool)
  n34 = global read "Globals.vi" "write to disc"() -> (w102:bool)
  n35 = global read "Globals.vi" "write to disc"() -> (w18:bool)
  n36 = global read "Globals.vi" "use ec cam"() -> (w362:bool)
  n37 = global read "Globals.vi" "use ec cam"() -> (w278:bool)
  n38 = global read "Globals.vi" "use ec cam"() -> (w190:bool)
  n39 = global read "Globals.vi" "use ec cam"() -> (w106:bool)
  n40 = global read "Globals.vi" "use ec cam"() -> (w22:bool)
  n41 = global read "Globals.vi" "btime[ms]"() -> (w422:dbl)
  n42 = global read "Globals.vi" "btime[ms]"() -> (w338:dbl)
  n43 = global read "Globals.vi" "btime[ms]"() -> (w250:dbl)
  n44 = global read "Globals.vi" "btime[ms]"() -> (w166:dbl)
  n45 = global read "Globals.vi" "btime[ms]"() -> (w82:dbl)
  n46 = global read "Globals.vi" "IS HS IR"() -> (w388:bool)
  n47 = global read "Globals.vi" "IS HS IR"() -> (w304:bool)
  n48 = global read "Globals.vi" "IS HS IR"() -> (w216:bool)
  n49 = global read "Globals.vi" "IS HS IR"() -> (w132:bool)
  n50 = global read "Globals.vi" "IS HS IR"() -> (w48:bool)
  n51 = global read "Globals.vi" "shortrs"() -> (w361:bool)
  n52 = global read "Globals.vi" "shortrs"() -> (w277:bool)
  n53 = global read "Globals.vi" "shortrs"() -> (w189:bool)
  n54 = global read "Globals.vi" "shortrs"() -> (w105:bool)
  n55 = global read "Globals.vi" "shortrs"() -> (w21:bool)
  n56 = global read "Globals.vi" "mshut"() -> (w406:bool)
  n57 = global read "Globals.vi" "led off"() -> (w402:bool)
  n58 = global read "Globals.vi" "mshut"() -> (w322:bool)
  n59 = global read "Globals.vi" "led off"() -> (w318:bool)
  n60 = global read "Globals.vi" "mshut"() -> (w234:bool)
  n61 = global read "Globals.vi" "led off"() -> (w230:bool)
  n62 = global read "Globals.vi" "mshut"() -> (w150:bool)
  n63 = global read "Globals.vi" "led off"() -> (w146:bool)
  n64 = global read "Globals.vi" "mshut"() -> (w66:bool)
  n65 = global read "Globals.vi" "led off"() -> (w62:bool)
  n66 = Multiply(x=w425, y=1000.0) -> (x*y=w424:dbl)
  n67 = Multiply(x=w341, y=1000.0) -> (x*y=w340:dbl)
  n68 = Multiply(x=w253, y=1000.0) -> (x*y=w252:dbl)
  n69 = Multiply(x=w169, y=1000.0) -> (x*y=w168:dbl)
  n70 = Multiply(x=w85, y=1000.0) -> (x*y=w84:dbl)
  n71 = global read "Globals.vi" "FFT"() -> (w412:bool)
  n72 = global read "Globals.vi" "FFT"() -> (w328:bool)
  n73 = global read "Globals.vi" "FFT"() -> (w240:bool)
  n74 = global read "Globals.vi" "FFT"() -> (w156:bool)
  n75 = global read "Globals.vi" "FFT"() -> (w72:bool)
  n76 = Initialize Array(u8 0 ("element"), 256 ("dimension size")) -> (w352:u8[])
  n77 = Initialize Array(u8 0 ("element"), 256 ("dimension size")) -> (w268:u8[])
  n78 = Initialize Array(u8 0 ("element"), 256 ("dimension size")) -> (w180:u8[])
  n79 = Initialize Array(u8 0 ("element"), 256 ("dimension size")) -> (w96:u8[])
  n80 = Initialize Array(u8 0 ("element"), 256 ("dimension size")) -> (w12:u8[])
  n81 = global read "Globals.vi" "ioctrl out width[5ns]"() -> (w372:u32[])
  n82 = global read "Globals.vi" "ioctrl out width[5ns]"() -> (w288:u32[])
  n83 = global read "Globals.vi" "ioctrl out width[5ns]"() -> (w200:u32[])
  n84 = global read "Globals.vi" "ioctrl out width[5ns]"() -> (w116:u32[])
  n85 = global read "Globals.vi" "ioctrl out width[5ns]"() -> (w32:u32[])
  n86 = global read "Globals.vi" "ioctrl out delay[5ns]"() -> (w375:u32[])
  n87 = global read "Globals.vi" "ioctrl out delay[5ns]"() -> (w291:u32[])
  n88 = global read "Globals.vi" "ioctrl out delay[5ns]"() -> (w203:u32[])
  n89 = global read "Globals.vi" "ioctrl out delay[5ns]"() -> (w119:u32[])
  n90 = global read "Globals.vi" "ioctrl out delay[5ns]"() -> (w35:u32[])
  n91 = Replace Array Subset(array=w352, new element=w350, index=0) -> (w349:u8[])
  n92 = Replace Array Subset(array=w268, new element=w266, index=0) -> (w265:u8[])
  n93 = Replace Array Subset(array=w180, new element=w178, index=0) -> (w177:u8[])
  n94 = Replace Array Subset(array=w96, new element=w94, index=0) -> (w93:u8[])
  n95 = Replace Array Subset(array=w12, new element=w10, index=0) -> (w9:u8[])
  n96 = global read "Globals.vi" "dac board1"() -> (w383:u32[])
  n97 = global read "Globals.vi" "dac board2"() -> (w299:u32[])
  n98 = global read "Globals.vi" "dac board3"() -> (w211:u32[])
  n99 = global read "Globals.vi" "dac board4"() -> (w127:u32[])
  n100 = global read "Globals.vi" "dac board5"() -> (w43:u32[])
  n101 = Boolean To (0,1)(Boolean=w414) -> (0, 1=w369:i16)
  n102 = To Unsigned Long Integer(number=w424) -> (unsigned 32bit integer=w391:u32)
  n103 = Boolean To (0,1)(Boolean=w412) -> (0, 1=w410:i16)
  n104 = Boolean To (0,1)(Boolean=w330) -> (0, 1=w285:i16)
  n105 = To Unsigned Long Integer(number=w340) -> (unsigned 32bit integer=w307:u32)
  n106 = Boolean To (0,1)(Boolean=w406) -> (0, 1=w405:i16)
  n107 = Boolean To (0,1)(Boolean=w402) -> (0, 1=w403:i16)
  n108 = Boolean To (0,1)(Boolean=w361) -> (0, 1=w360:i16)
  n109 = Boolean To (0,1)(Boolean=w328) -> (0, 1=w326:i16)
  n110 = Boolean To (0,1)(Boolean=w242) -> (0, 1=w197:i16)
  n111 = To Unsigned Long Integer(number=w252) -> (unsigned 32bit integer=w219:u32)
  n112 = Boolean To (0,1)(Boolean=w322) -> (0, 1=w321:i16)
  n113 = global read "Globals.vi" "region size"() -> (w386:u32[])
  n114 = Boolean To (0,1)(Boolean=w318) -> (0, 1=w319:i16)
  n115 = Boolean To (0,1)(Boolean=w277) -> (0, 1=w276:i16)
  n116 = Boolean To (0,1)(Boolean=w388) -> (0, 1=w387:i16)
  n117 = Boolean To (0,1)(Boolean=w240) -> (0, 1=w238:i16)
  n118 = Boolean To (0,1)(Boolean=w158) -> (0, 1=w113:i16)
  n119 = To Unsigned Long Integer(number=w168) -> (unsigned 32bit integer=w135:u32)
  n120 = Boolean To (0,1)(Boolean=w234) -> (0, 1=w233:i16)
  n121 = global read "Globals.vi" "region size"() -> (w302:u32[])
  n122 = Boolean To (0,1)(Boolean=w230) -> (0, 1=w231:i16)
  n123 = Boolean To (0,1)(Boolean=w362) -> (0, 1=w364:i16)
  n124 = Boolean To (0,1)(Boolean=w358) -> (0, 1=w359:i16)
  n125 = Boolean To (0,1)(Boolean=w189) -> (0, 1=w188:i16)
  n126 = Boolean To (0,1)(Boolean=w347) -> (0, 1=w346:i16)
  n127 = Boolean To (0,1)(Boolean=w304) -> (0, 1=w303:i16)
  n128 = Boolean To (0,1)(Boolean=w156) -> (0, 1=w154:i16)
  n129 = Boolean To (0,1)(Boolean=w74) -> (0, 1=w29:i16)
  n130 = To Unsigned Long Integer(number=w84) -> (unsigned 32bit integer=w51:u32)
  n131 = Boolean To (0,1)(Boolean=w150) -> (0, 1=w149:i16)
  n132 = global read "Globals.vi" "region size"() -> (w214:u32[])
  n133 = Boolean To (0,1)(Boolean=w146) -> (0, 1=w147:i16)
  n134 = Boolean To (0,1)(Boolean=w278) -> (0, 1=w280:i16)
  n135 = Boolean To (0,1)(Boolean=w274) -> (0, 1=w275:i16)
  n136 = Boolean To (0,1)(Boolean=w105) -> (0, 1=w104:i16)
  n137 = Boolean To (0,1)(Boolean=w263) -> (0, 1=w262:i16)
  n138 = Boolean To (0,1)(Boolean=w216) -> (0, 1=w215:i16)
  n139 = Boolean To (0,1)(Boolean=w72) -> (0, 1=w70:i16)
  n140 = Boolean To (0,1)(Boolean=w66) -> (0, 1=w65:i16)
  n141 = global read "Globals.vi" "region size"() -> (w130:u32[])
  n142 = Boolean To (0,1)(Boolean=w62) -> (0, 1=w63:i16)
  n143 = Boolean To (0,1)(Boolean=w190) -> (0, 1=w192:i16)
  n144 = Boolean To (0,1)(Boolean=w186) -> (0, 1=w187:i16)
  n145 = Boolean To (0,1)(Boolean=w21) -> (0, 1=w20:i16)
  n146 = Boolean To (0,1)(Boolean=w175) -> (0, 1=w174:i16)
  n147 = Boolean To (0,1)(Boolean=w132) -> (0, 1=w131:i16)
  n148 = global read "Globals.vi" "region size"() -> (w46:u32[])
  n149 = Boolean To (0,1)(Boolean=w106) -> (0, 1=w108:i16)
  n150 = Boolean To (0,1)(Boolean=w102) -> (0, 1=w103:i16)
  n151 = Boolean To (0,1)(Boolean=w91) -> (0, 1=w90:i16)
  n152 = Boolean To (0,1)(Boolean=w48) -> (0, 1=w47:i16)
  n153 = Boolean To (0,1)(Boolean=w22) -> (0, 1=w24:i16)
  n154 = Boolean To (0,1)(Boolean=w18) -> (0, 1=w19:i16)
  n155 = Boolean To (0,1)(Boolean=w7) -> (0, 1=w6:i16)
  n156 = Multiply(x=w422, y=1000.0) -> (x*y=w421:dbl)
  n157 = Multiply(x=w338, y=1000.0) -> (x*y=w337:dbl)
  n158 = Multiply(x=w250, y=1000.0) -> (x*y=w249:dbl)
  n159 = Multiply(x=w166, y=1000.0) -> (x*y=w165:dbl)
  n160 = Multiply(x=w82, y=1000.0) -> (x*y=w81:dbl)
  n161 = global read "Globals.vi" "continuous"() -> (w258:bool)
  n162 = To Unsigned Long Integer(number=w369) -> (unsigned 32bit integer=w368:u32)
  n163 = To Unsigned Long Integer(number=w421) -> (unsigned 32bit integer=w419:u32)
  n164 = To Unsigned Long Integer(number=w410) -> (unsigned 32bit integer=w411:u32)
  n165 = To Unsigned Long Integer(number=w285) -> (unsigned 32bit integer=w284:u32)
  n166 = To Unsigned Long Integer(number=w405) -> (unsigned 32bit integer=w404:u32)
  n167 = To Unsigned Long Integer(number=w337) -> (unsigned 32bit integer=w335:u32)
  n168 = To Unsigned Long Integer(number=w403) -> (unsigned 32bit integer=w401:u32)
  n169 = To Unsigned Long Integer(number=w360) -> (unsigned 32bit integer=w398:u32)
  n170 = To Unsigned Long Integer(number=w326) -> (unsigned 32bit integer=w327:u32)
  n171 = To Unsigned Long Integer(number=w197) -> (unsigned 32bit integer=w196:u32)
  n172 = To Unsigned Long Integer(number=w321) -> (unsigned 32bit integer=w320:u32)
  n173 = To Unsigned Long Integer(number=w249) -> (unsigned 32bit integer=w247:u32)
  n174 = To Unsigned Long Integer(number=w319) -> (unsigned 32bit integer=w317:u32)
  n175 = To Unsigned Long Integer(number=w276) -> (unsigned 32bit integer=w314:u32)
  n176 = To Unsigned Long Integer(number=w387) -> (unsigned 32bit integer=w379:u32)
  n177 = To Unsigned Long Integer(number=w238) -> (unsigned 32bit integer=w239:u32)
  n178 = To Unsigned Long Integer(number=w113) -> (unsigned 32bit integer=w112:u32)
  n179 = To Unsigned Long Integer(number=w233) -> (unsigned 32bit integer=w232:u32)
  n180 = To Unsigned Long Integer(number=w165) -> (unsigned 32bit integer=w163:u32)
  n181 = To Unsigned Long Integer(number=w231) -> (unsigned 32bit integer=w229:u32)
  n182 = To Unsigned Long Integer(number=w364) -> (unsigned 32bit integer=w363:u32)
  n183 = To Unsigned Long Integer(number=w359) -> (unsigned 32bit integer=w357:u32)
  n184 = To Unsigned Long Integer(number=w188) -> (unsigned 32bit integer=w226:u32)
  n185 = To Unsigned Long Integer(number=w346) -> (unsigned 32bit integer=w345:u32)
  n186 = To Unsigned Long Integer(number=w303) -> (unsigned 32bit integer=w295:u32)
  n187 = To Unsigned Long Integer(number=w154) -> (unsigned 32bit integer=w155:u32)
  n188 = To Unsigned Long Integer(number=w29) -> (unsigned 32bit integer=w28:u32)
  n189 = To Unsigned Long Integer(number=w149) -> (unsigned 32bit integer=w148:u32)
  n190 = To Unsigned Long Integer(number=w81) -> (unsigned 32bit integer=w79:u32)
  n191 = To Unsigned Long Integer(number=w147) -> (unsigned 32bit integer=w145:u32)
  n192 = To Unsigned Long Integer(number=w280) -> (unsigned 32bit integer=w279:u32)
  n193 = To Unsigned Long Integer(number=w275) -> (unsigned 32bit integer=w273:u32)
  n194 = To Unsigned Long Integer(number=w104) -> (unsigned 32bit integer=w142:u32)
  n195 = To Unsigned Long Integer(number=w262) -> (unsigned 32bit integer=w261:u32)
  n196 = To Unsigned Long Integer(number=w215) -> (unsigned 32bit integer=w207:u32)
  n197 = To Unsigned Long Integer(number=w70) -> (unsigned 32bit integer=w71:u32)
  n198 = To Unsigned Long Integer(number=w65) -> (unsigned 32bit integer=w64:u32)
  n199 = To Unsigned Long Integer(number=w63) -> (unsigned 32bit integer=w61:u32)
  n200 = To Unsigned Long Integer(number=w192) -> (unsigned 32bit integer=w191:u32)
  n201 = To Unsigned Long Integer(number=w187) -> (unsigned 32bit integer=w185:u32)
  n202 = To Unsigned Long Integer(number=w20) -> (unsigned 32bit integer=w58:u32)
  n203 = To Unsigned Long Integer(number=w174) -> (unsigned 32bit integer=w173:u32)
  n204 = To Unsigned Long Integer(number=w131) -> (unsigned 32bit integer=w123:u32)
  n205 = To Unsigned Long Integer(number=w108) -> (unsigned 32bit integer=w107:u32)
  n206 = To Unsigned Long Integer(number=w103) -> (unsigned 32bit integer=w101:u32)
  n207 = To Unsigned Long Integer(number=w90) -> (unsigned 32bit integer=w89:u32)
  n208 = To Unsigned Long Integer(number=w47) -> (unsigned 32bit integer=w39:u32)
  n209 = To Unsigned Long Integer(number=w24) -> (unsigned 32bit integer=w23:u32)
  n210 = To Unsigned Long Integer(number=w19) -> (unsigned 32bit integer=w17:u32)
  n211 = To Unsigned Long Integer(number=w6) -> (unsigned 32bit integer=w5:u32)
  n212 = Array To Cluster(array=w386) -> (cluster=w385:T1)
  n213 = Array To Cluster(array=w383) -> (cluster=w384:T2)
  n214 = Array To Cluster(array=w372) -> (cluster=w376:T3)
  n215 = Array To Cluster(array=w375) -> (cluster=w374:T4)
  n216 = Array To Cluster(array=w302) -> (cluster=w301:T1)
  n217 = Array To Cluster(array=w299) -> (cluster=w300:T5)
  n218 = Array To Cluster(array=w349) -> (cluster=w348:T6)
  n219 = Array To Cluster(array=w288) -> (cluster=w292:T3)
  n220 = Array To Cluster(array=w291) -> (cluster=w290:T4)
  n221 = Array To Cluster(array=w214) -> (cluster=w213:T1)
  n222 = Array To Cluster(array=w211) -> (cluster=w212:T7)
  n223 = Array To Cluster(array=w265) -> (cluster=w264:T6)
  n224 = Array To Cluster(array=w200) -> (cluster=w204:T3)
  n225 = Array To Cluster(array=w203) -> (cluster=w202:T4)
  n226 = Array To Cluster(array=w130) -> (cluster=w129:T1)
  n227 = Array To Cluster(array=w127) -> (cluster=w128:T8)
  n228 = Array To Cluster(array=w177) -> (cluster=w176:T6)
  n229 = Array To Cluster(array=w116) -> (cluster=w120:T3)
  n230 = Array To Cluster(array=w119) -> (cluster=w118:T4)
  n231 = Array To Cluster(array=w46) -> (cluster=w45:T1)
  n232 = Array To Cluster(array=w43) -> (cluster=w44:T9)
  n233 = Array To Cluster(array=w93) -> (cluster=w92:T6)
  n234 = Array To Cluster(array=w32) -> (cluster=w36:T3)
  n235 = Array To Cluster(array=w35) -> (cluster=w34:T4)
  n236 = Array To Cluster(array=w9) -> (cluster=w8:T6)
  n237 = global read "Globals.vi" "dma buffer size in scans"() -> (w367:u32)
  n238 = global read "Globals.vi" "dma buffer size in scans"() -> (w283:u32)
  n239 = global read "Globals.vi" "dma buffer size in scans"() -> (w195:u32)
  n240 = global read "Globals.vi" "dma buffer size in scans"() -> (w111:u32)
  n241 = global read "Globals.vi" "dma buffer size in scans"() -> (w27:u32)
  n242 = global read "Globals.vi" "ioctrl impact start pixel"() -> (w377:u32)
  n243 = global read "Globals.vi" "ioctrl impact start pixel"() -> (w293:u32)
  n244 = global read "Globals.vi" "ioctrl impact start pixel"() -> (w205:u32)
  n245 = global read "Globals.vi" "ioctrl impact start pixel"() -> (w121:u32)
  n246 = global read "Globals.vi" "ioctrl impact start pixel"() -> (w37:u32)
  n247 = global read "Globals.vi" "ioctrl t0 period[10ns]"() -> (w373:u32)
  n248 = global read "Globals.vi" "ioctrl t0 period[10ns]"() -> (w289:u32)
  n249 = global read "Globals.vi" "ioctrl t0 period[10ns]"() -> (w201:u32)
  n250 = global read "Globals.vi" "ioctrl t0 period[10ns]"() -> (w117:u32)
  n251 = global read "Globals.vi" "ioctrl t0 period[10ns]"() -> (w33:u32)
  n252 = global read "Globals.vi" "CAMERA SYSTEM"() -> (w409:u32)
  n253 = global read "Globals.vi" "area lines binning"() -> (w393:u32)
  n254 = global read "Globals.vi" "CAMERA SYSTEM"() -> (w325:u32)
  n255 = global read "Globals.vi" "CAMERA SYSTEM"() -> (w237:u32)
  n256 = global read "Globals.vi" "area lines binning"() -> (w309:u32)
  n257 = global read "Globals.vi" "area lines binning"() -> (w221:u32)
  n258 = global read "Globals.vi" "CAMERA SYSTEM"() -> (w153:u32)
  n259 = global read "Globals.vi" "area lines binning"() -> (w137:u32)
  n260 = global read "Globals.vi" "CAMERA SYSTEM"() -> (w69:u32)
  n261 = global read "Globals.vi" "area lines binning"() -> (w53:u32)
  n262 = global read "Globals.vi" "custom pattern"() -> (w381:u32)
  n263 = global read "Globals.vi" "custom pattern"() -> (w297:u32)
  n264 = global read "Globals.vi" "custom pattern"() -> (w209:u32)
  n265 = global read "Globals.vi" "custom pattern"() -> (w125:u32)
  n266 = global read "Globals.vi" "custom pattern"() -> (w41:u32)
  n267 = global read "Globals.vi" "xckdly in 10ns"() -> (w390:u32)
  n268 = global read "Globals.vi" "xckdly in 10ns"() -> (w306:u32)
  n269 = global read "Globals.vi" "xckdly in 10ns"() -> (w218:u32)
  n270 = global read "Globals.vi" "xckdly in 10ns"() -> (w134:u32)
  n271 = global read "Globals.vi" "xckdly in 10ns"() -> (w50:u32)
  n272 = Boolean To (0,1)(Boolean=w258) -> (0, 1=w257:i16)
  n273 = global read "Globals.vi" "bdat in 10ns"() -> (w417:u32)
  n274 = global read "Globals.vi" "bdat in 10ns"() -> (w333:u32)
  n275 = global read "Globals.vi" "bdat in 10ns"() -> (w245:u32)
  n276 = global read "Globals.vi" "bdat in 10ns"() -> (w161:u32)
  n277 = global read "Globals.vi" "bdat in 10ns"() -> (w77:u32)
  n278 = global read "Globals.vi" "sdat in 10ns"() -> (w418:u32)
  n279 = global read "Globals.vi" "sdat in 10ns"() -> (w334:u32)
  n280 = global read "Globals.vi" "bec in 10\nns"() -> (w380:u32)
  n281 = global read "Globals.vi" "sdat in 10ns"() -> (w246:u32)
  n282 = global read "Globals.vi" "bec in 10\nns"() -> (w296:u32)
  n283 = global read "Globals.vi" "sdat in 10ns"() -> (w162:u32)
  n284 = global read "Globals.vi" "bec in 10\nns"() -> (w208:u32)
  n285 = global read "Globals.vi" "sdat in 10ns"() -> (w78:u32)
  n286 = global read "Globals.vi" "bec in 10\nns"() -> (w124:u32)
  n287 = global read "Globals.vi" "bec in 10\nns"() -> (w40:u32)
  n288 = global read "Globals.vi" "sensor gain"() -> (w370:u32)
  n289 = global read "Globals.vi" "sensor gain"() -> (w286:u32)
  n290 = global read "Globals.vi" "sensor gain"() -> (w198:u32)
  n291 = global read "Globals.vi" "sensor gain"() -> (w114:u32)
  n292 = global read "Globals.vi" "sensor gain"() -> (w30:u32)
  n293 = global read "Globals.vi" "sec in 10ns"() -> (w389:u32)
  n294 = global read "Globals.vi" "sec in 10ns"() -> (w305:u32)
  n295 = global read "Globals.vi" "sec in 10ns"() -> (w217:u32)
  n296 = global read "Globals.vi" "sec in 10ns"() -> (w133:u32)
  n297 = global read "Globals.vi" "sec in 10ns"() -> (w49:u32)
  n298 = global read "Globals.vi" "gpx offset"() -> (w397:u32)
  n299 = global read "Globals.vi" "adc mode"() -> (w382:enum16{"normal", "ramp", "custom pattern"})
  n300 = global read "Globals.vi" "gpx offset"() -> (w313:u32)
  n301 = global read "Globals.vi" "adc mode"() -> (w298:enum16{"normal", "ramp", "custom pattern"})
  n302 = global read "Globals.vi" "gpx offset"() -> (w225:u32)
  n303 = global read "Globals.vi" "adc mode"() -> (w210:enum16{"normal", "ramp", "custom pattern"})
  n304 = global read "Globals.vi" "gpx offset"() -> (w141:u32)
  n305 = global read "Globals.vi" "adc mode"() -> (w126:enum16{"normal", "ramp", "custom pattern"})
  n306 = global read "Globals.vi" "gpx offset"() -> (w57:u32)
  n307 = global read "Globals.vi" "adc mode"() -> (w42:enum16{"normal", "ramp", "custom pattern"})
  n308 = global read "Globals.vi" "cc trigger"() -> (w413:enum32{"XCK", "Ext. Trig.", "DAT"})
  n309 = global read "Globals.vi" "CAMCNT"() -> (w408:u32)
  n310 = global read "Globals.vi" "cool level"() -> (w399:u32)
  n311 = global read "Globals.vi" "cc trigger"() -> (w329:enum32{"XCK", "Ext. Trig.", "DAT"})
  n312 = global read "Globals.vi" "CAMCNT"() -> (w324:u32)
  n313 = global read "Globals.vi" "cool level"() -> (w315:u32)
  n314 = global read "Globals.vi" "cc trigger"() -> (w241:enum32{"XCK", "Ext. Trig.", "DAT"})
  n315 = global read "Globals.vi" "CAMCNT"() -> (w236:u32)
  n316 = global read "Globals.vi" "cool level"() -> (w227:u32)
  n317 = global read "Globals.vi" "cc trigger"() -> (w157:enum32{"XCK", "Ext. Trig.", "DAT"})
  n318 = global read "Globals.vi" "CAMCNT"() -> (w152:u32)
  n319 = global read "Globals.vi" "cool level"() -> (w143:u32)
  n320 = global read "Globals.vi" "cc trigger"() -> (w73:enum32{"XCK", "Ext. Trig.", "DAT"})
  n321 = global read "Globals.vi" "CAMCNT"() -> (w68:u32)
  n322 = global read "Globals.vi" "cool level"() -> (w59:u32)
  n323 = global read "Globals.vi" "adc gain"() -> (w400:u32)
  n324 = global read "Globals.vi" "fft mode"() -> (w394:T10)
  n325 = global read "Globals.vi" "adc gain"() -> (w316:u32)
  n326 = global read "Globals.vi" "fft mode"() -> (w310:T10)
  n327 = global read "Globals.vi" "adc gain"() -> (w228:u32)
  n328 = global read "Globals.vi" "fft mode"() -> (w222:T10)
  n329 = global read "Globals.vi" "adc gain"() -> (w144:u32)
  n330 = global read "Globals.vi" "fft mode"() -> (w138:T10)
  n331 = global read "Globals.vi" "adc gain"() -> (w60:u32)
  n332 = global read "Globals.vi" "fft mode"() -> (w54:T10)
  n333 = global read "Globals.vi" "bt slope"() -> (w415:enum32{"neg", "pos", "both"})
  n334 = global read "Globals.vi" "bt slope"() -> (w331:enum32{"neg", "pos", "both"})
  n335 = global read "Globals.vi" "bt slope"() -> (w243:enum32{"neg", "pos", "both"})
  n336 = global read "Globals.vi" "bt slope"() -> (w159:enum32{"neg", "pos", "both"})
  n337 = global read "Globals.vi" "bt slope"() -> (w75:enum32{"neg", "pos", "both"})
  n338 = global read "Globals.vi" "st slope"() -> (w416:enum32{"pos", "neg", "both"})
  n339 = global read "Globals.vi" "st slope"() -> (w332:enum32{"pos", "neg", "both"})
  n340 = global read "Globals.vi" "st slope"() -> (w244:enum32{"pos", "neg", "both"})
  n341 = global read "Globals.vi" "st slope"() -> (w160:enum32{"pos", "neg", "both"})
  n342 = global read "Globals.vi" "st slope"() -> (w76:enum32{"pos", "neg", "both"})
  n343 = global read "Globals.vi" "VFREQ"() -> (w395:u32)
  n344 = global read "Globals.vi" "VFREQ"() -> (w311:u32)
  n345 = global read "Globals.vi" "VFREQ"() -> (w223:u32)
  n346 = global read "Globals.vi" "VFREQ"() -> (w139:u32)
  n347 = global read "Globals.vi" "VFREQ"() -> (w55:u32)
  n348 = global read "Globals.vi" "PIXEL"() -> (w407:u32)
  n349 = global read "Globals.vi" "LINES"() -> (w396:u32)
  n350 = global read "Globals.vi" "PIXEL"() -> (w323:u32)
  n351 = global read "Globals.vi" "LINES"() -> (w312:u32)
  n352 = global read "Globals.vi" "PIXEL"() -> (w235:u32)
  n353 = global read "Globals.vi" "LINES"() -> (w224:u32)
  n354 = global read "Globals.vi" "PIXEL"() -> (w151:u32)
  n355 = global read "Globals.vi" "LINES"() -> (w140:u32)
  n356 = global read "Globals.vi" "PIXEL"() -> (w67:u32)
  n357 = global read "Globals.vi" "LINES"() -> (w56:u32)
  n358 = global read "Globals.vi" "tocnt"() -> (w366:u32)
  n359 = global read "Globals.vi" "tocnt"() -> (w282:u32)
  n360 = global read "Globals.vi" "tocnt"() -> (w194:u32)
  n361 = global read "Globals.vi" "tocnt"() -> (w110:u32)
  n362 = global read "Globals.vi" "tocnt"() -> (w26:u32)
  n363 = global read "Globals.vi" "ticnt"() -> (w365:u32)
  n364 = global read "Globals.vi" "ticnt"() -> (w281:u32)
  n365 = global read "Globals.vi" "ticnt"() -> (w193:u32)
  n366 = global read "Globals.vi" "ticnt"() -> (w109:u32)
  n367 = global read "Globals.vi" "ticnt"() -> (w25:u32)
  n368 = global read "Globals.vi" "nor"() -> (w392:u32)
  n369 = global read "Globals.vi" "nor"() -> (w308:u32)
  n370 = global read "Globals.vi" "nor"() -> (w220:u32)
  n371 = global read "Globals.vi" "nor"() -> (w136:u32)
  n372 = global read "Globals.vi" "nor"() -> (w52:u32)
  n373 = global read "Globals.vi" "tor"() -> (w378:T11)
  n374 = global read "Globals.vi" "tor"() -> (w294:T11)
  n375 = global read "Globals.vi" "tor"() -> (w206:T11)
  n376 = global read "Globals.vi" "tor"() -> (w122:T11)
  n377 = global read "Globals.vi" "tor"() -> (w38:T11)
  n378 = global read "Globals.vi" "bti"() -> (w426:T12)
  n379 = global read "Globals.vi" "bti"() -> (w342:T12)
  n380 = global read "Globals.vi" "bti"() -> (w254:T12)
  n381 = global read "Globals.vi" "bti"() -> (w170:T12)
  n382 = global read "Globals.vi" "bti"() -> (w86:T12)
  n383 = global read "Globals.vi" "sti"() -> (w427:T13)
  n384 = global read "Globals.vi" "sti"() -> (w343:T13)
  n385 = global read "Globals.vi" "sti"() -> (w255:T13)
  n386 = global read "Globals.vi" "sti"() -> (w171:T13)
  n387 = global read "Globals.vi" "sti"() -> (w87:T13)
  n388 = Bundle "camera settings board 0"(w368, "sti"=w427, "bti"=w426, w391, w419, "sdat in 10ns"=w418, "bdat in 10ns"=w417, "st slope"=w416, "bt slope"=w415, "xckdly in 10ns"=w390, "sec in 10ns"=w389, "cc trigger"=w413, w411, "CAMERA SYSTEM"=w409, "CAMCNT"=w408, "PIXEL"=w407, w404, w401, "sensor gain"=w370, "adc gain"=w400, "cool level"=w399, w398, "gpx offset"=w397, "LINES"=w396, "VFREQ"=w395, "fft mode"=w394, "area lines binning"=w393, "nor"=w392, u8 255, "region size"=w385, "dac board1"=w384, "tor"=w378, "adc mode"=w382, "custom pattern"=w381, "bec in 10\nns"=w380, w379, "ioctrl impact start pixel"=w377, "ioctrl out width[5ns]"=w376, "ioctrl out delay[5ns]"=w374, "ioctrl t0 period[10ns]"=w373, "dma buffer size in scans"=w367, "tocnt"=w366, "ticnt"=w365, w363, w357, w348, "unused (deprecated file split mode)"=w344, w345) -> (w430:T14)  [unwired: 1 in]
  n389 = Bundle "camera settings board 1"(w284, "sti"=w343, "bti"=w342, w307, w335, "sdat in 10ns"=w334, "bdat in 10ns"=w333, "st slope"=w332, "bt slope"=w331, "xckdly in 10ns"=w306, "sec in 10ns"=w305, "cc trigger"=w329, w327, "CAMERA SYSTEM"=w325, "CAMCNT"=w324, "PIXEL"=w323, w320, w317, "sensor gain"=w286, "adc gain"=w316, "cool level"=w315, w314, "gpx offset"=w313, "LINES"=w312, "VFREQ"=w311, "fft mode"=w310, "area lines binning"=w309, "nor"=w308, u8 255, "region size"=w301, "dac board2"=w300, "tor"=w294, "adc mode"=w298, "custom pattern"=w297, "bec in 10\nns"=w296, w295, "ioctrl impact start pixel"=w293, "ioctrl out width[5ns]"=w292, "ioctrl out delay[5ns]"=w290, "ioctrl t0 period[10ns]"=w289, "dma buffer size in scans"=w283, "tocnt"=w282, "ticnt"=w281, w279, w273, w264, "unused (deprecated file split mode)"=w260, w261) -> (w259:T15)  [unwired: 1 in]
  n390 = Bundle "camera settings board 2"(w196, "sti"=w255, "bti"=w254, w219, w247, "sdat in 10ns"=w246, "bdat in 10ns"=w245, "st slope"=w244, "bt slope"=w243, "xckdly in 10ns"=w218, "sec in 10ns"=w217, "cc trigger"=w241, w239, "CAMERA SYSTEM"=w237, "CAMCNT"=w236, "PIXEL"=w235, w232, w229, "sensor gain"=w198, "adc gain"=w228, "cool level"=w227, w226, "gpx offset"=w225, "LINES"=w224, "VFREQ"=w223, "fft mode"=w222, "area lines binning"=w221, "nor"=w220, u8 255, "region size"=w213, "dac board3"=w212, "tor"=w206, "adc mode"=w210, "custom pattern"=w209, "bec in 10\nns"=w208, w207, "ioctrl impact start pixel"=w205, "ioctrl out width[5ns]"=w204, "ioctrl out delay[5ns]"=w202, "ioctrl t0 period[10ns]"=w201, "dma buffer size in scans"=w195, "tocnt"=w194, "ticnt"=w193, w191, w185, w176, "unused (deprecated file split mode)"=w172, w173) -> (w3:T16)  [unwired: 1 in]
  n391 = Bundle "camera settings board 3"(w112, "sti"=w171, "bti"=w170, w135, w163, "sdat in 10ns"=w162, "bdat in 10ns"=w161, "st slope"=w160, "bt slope"=w159, "xckdly in 10ns"=w134, "sec in 10ns"=w133, "cc trigger"=w157, w155, "CAMERA SYSTEM"=w153, "CAMCNT"=w152, "PIXEL"=w151, w148, w145, "sensor gain"=w114, "adc gain"=w144, "cool level"=w143, w142, "gpx offset"=w141, "LINES"=w140, "VFREQ"=w139, "fft mode"=w138, "area lines binning"=w137, "nor"=w136, u8 255, "region size"=w129, "dac board4"=w128, "tor"=w122, "adc mode"=w126, "custom pattern"=w125, "bec in 10\nns"=w124, w123, "ioctrl impact start pixel"=w121, "ioctrl out width[5ns]"=w120, "ioctrl out delay[5ns]"=w118, "ioctrl t0 period[10ns]"=w117, "dma buffer size in scans"=w111, "tocnt"=w110, "ticnt"=w109, w107, w101, w92, "unused (deprecated file split mode)"=w88, w89) -> (w2:T17)  [unwired: 1 in]
  n392 = Bundle "camera settings board 4"(w28, "sti"=w87, "bti"=w86, w51, w79, "sdat in 10ns"=w78, "bdat in 10ns"=w77, "st slope"=w76, "bt slope"=w75, "xckdly in 10ns"=w50, "sec in 10ns"=w49, "cc trigger"=w73, w71, "CAMERA SYSTEM"=w69, "CAMCNT"=w68, "PIXEL"=w67, w64, w61, "sensor gain"=w30, "adc gain"=w60, "cool level"=w59, w58, "gpx offset"=w57, "LINES"=w56, "VFREQ"=w55, "fft mode"=w54, "area lines binning"=w53, "nor"=w52, u8 255, "region size"=w45, "dac board5"=w44, "tor"=w38, "adc mode"=w42, "custom pattern"=w41, "bec in 10\nns"=w40, w39, "ioctrl impact start pixel"=w37, "ioctrl out width[5ns]"=w36, "ioctrl out delay[5ns]"=w34, "ioctrl t0 period[10ns]"=w33, "dma buffer size in scans"=w27, "tocnt"=w26, "ticnt"=w25, w23, w17, w8, "unused (deprecated file split mode)"=w4, w5) -> (w1:T18)  [unwired: 1 in]
  n393 = To Unsigned Long Integer(number=w257) -> (unsigned 32bit integer=w256:u32)
  n394 = global read "Globals.vi" "cont pause in microseconds"() -> (w428:u32)
  n395 = global read "Globals.vi" "board_sel"() -> (w433:u32)
  n396 = global read "Globals.vi" "nob"() -> (w431:u32)
  n397 = global read "Globals.vi" "nos"() -> (w432:u32)
  n398 = Bundle "measurement settings"("board_sel"=w433, "nos"=w432, "nob"=w431, w256, "cont pause in microseconds"=w428, w430, w259, w3, w2, w1) -> (w429:T19)  [unwired: 1 in]
  n399 = call <vilib>:"Application Directory.vi"() -> ("Application Directory"=w437:path)
  n400 = Build Path(base path=w437, name or relative path="board.vis\\ESLSCDLL.dll") -> (appended path=w435:path)
  n401 = dll-call lib="C:/ENTW/PCIE/LV64/board.vis/ESLSCDLL.dll" fn="DLLSetGlobalSettings" ("lwlscdll.dll:DLLSetISFFT")(path in=w435, error in="error in (no error)", "struct measurement_settings"=w429) -> (path out=w434:path, error out=w438:errorcluster)  [unwired: 3 in]
  n402 = dll-call lib="C:/ENTW/PCIE/LV64/board.vis/ESLSCDLL.dll" fn="DLLInitMeasurement" ("lwlscdll.dll:DLLSetISFFT")(path in=w434, error in=w438) -> (error out=w441:errorcluster, "es_status_codes"=w442:i32)  [unwired: 1 in, 1 out]
  n403 = call "Error Converter (ErrCode or Status).vi"("error in (no error)"=w441, "error code"=w442) -> ("error out"=→"error out":errorcluster)  [unwired: 9 in]
